vi "RoboIME_UI.vi"(9 "Com UDP":T14={"UDP GrSim TX"=TRUE, "Address:"="192.168.37.12", "Port:"=10301}, 10 "RefBox UDP RX":T13={"Local IP:"="", "Server IP:"="224.5.23.1", "Port"="10003"}, 11 "SSL UDP RX":T13={"Local IP:"="", "Server IP:"="224.5.23.2", "Port"="10020"}) -> ()   [LabVIEW 2022 SP3]
uses:
  Vision_class/Old vision/Controls/Estimadores.ctl
  Vision_class/Old vision/Decode SSL and Refree Wrapper Package Folder/SSL Referee Game Status.ctl
  Vision_class/Old vision/Draw Field Folder/DrawTargets.ctl
  Vision_class/Old vision/Controls/SSL Field State.ctl
  Vision_class/Old vision/Controls/SSL Detection Frame.ctl
  Vision_class/Old vision/Controls/SSL Detection Robot.ctl
  <vilib>/Analysis/Matrix/Datatypes/RealMatrix.ctl
  Vision_class/Old vision/Controls/SSL Detection Ball.ctl
  Communication_class/Communication.lvclass
  Controls/ComUDP.ctl
  Controls/ComSerial.ctl
  Controls/ComSOS.ctl
  Controls/PhoenixParameters.ctl
  Play_class/PassReceiver.ctl
  Parameters_class/ChoosePassReceiver.ctl
  Game_class/Navigation/Controls/bangBangControlParameters.ctl
  Parameters_class/Project.ctl
  Controls/RobotModelTestState.ctl
  Game_class/VelocityPlanningTest/Controls/testMode.ctl
  Controls/RobotModelReplacementTest.ctl
  Controls/grSimReplacement.ctl
  Communication_class/Paths/grSim Packet Command UDP Test Folder/grSim/grSim RobotReplacement.ctl
  Communication_class/Paths/grSim Packet Command UDP Test Folder/grSim/grSim_BallReplacement.ctl
  Game_class/KickValueTest/KickValuetest.ctl
  Game_class/KickValueTest/KickValue.ctl
  Game_class/KickValueTest/BallValue.ctl
  Game_class/VelocityPlanningTest/Controls/velocityPlanningState.ctl
  Game_class/VelocityPlanningTest/Controls/trajectoryState.ctl
  5RobotsPassGamePlay_class/PassFinishBallVelConditionDegub.ctl
  5RobotsPassGamePlay_class/PassFinishReceiverDistanceToBallConditionDebug.ctl
  Controls/Enviroment.ctl
  Team_class/KeeperPlay.ctl
  Team_class/OffensivePlay.ctl
  Referee_class/command_interpreted.ctl
  Robot_class/roles.ctl
  Robot_class/tactics.ctl
  Team_class/DefensivePlay.ctl
  Controls/vision_control.ctl
  Game_class/KickForceTest/Controls/kickForceTestState.ctl
  Game_class/KickForceTest/Controls/KickForceEnum.ctl
  Game_class/Replay/ReplayControls.ctl
  Game_class/ParametersFromFile/ParametersFromFile.ctl
  Robot_class/robotDisplayFeedback.ctl
  Controls/NewParameters.ctl
  Utilities_class/Style.ctl
  Vision_class/Vision.lvclass
  Game_class/Game.lvclass
  RobotFeedback/RobotFeedback.lvclass/RobotFeedback.ctl
  Game_class/Game.lvclass/Game.ctl
  Referee_class/Referee.lvclass/Referee.ctl
  Team_class/Team.lvclass/Team.ctl
  Robot_class/Robot.lvclass/Robot.ctl
  Game_class/ParametersFromFile/MainGameConfigs.ctl
  Robot_class/Robot.lvclass
  Events_class/Events.lvclass
  RobotFeedback/Read id.vi
  RobotFeedback/Read dribblerContactToBall.vi
  Game_class/Write RobotsFeedback.vi
  Robot_class/Read id.vi
  Robot_class/Read role.vi
  Robot_class/Read tactic.vi
  Game_class/Read Referee.vi
  Game_class/Read KeeperTeam.vi
  Game_class/Read OffensiveTeam.vi
  Game_class/Read DefensiveTeam.vi
  Team_class/Read RobotRef.vi
  Team_class/Read DefensivePlay.vi
  Team_class/Read OffensivePlay.vi
  Team_class/Read KeeperPlay.vi
  Referee_class/Read command_interpreted.vi
  Game_class/Write TestTeam.vi
  Game_class/Write DefensiveTeam.vi
  Game_class/Read AllyRef.vi
  Team_class/Write RobotRef.vi
  Game_class/Write NavigationTeam.vi
  Game_class/Write EventsRef.vi
  Game_class/Write OffensiveTeam.vi
  Game_class/Write KeeperTeam.vi
  Ally_class/Ally.lvclass
  C:/Users/ebert/Documents/codes/SSL/repo/SSL_AI/Team_class/Team.lvclass
  RobotFeedback/commCAS.vi
  Referee_class/Referee.lvclass
  Playbook_class/Playbook.lvclass
  <vilib>/Analysis/Matrix/NI_Matrix.lvlib
  RobotFeedback/RobotFeedback.lvclass
panel:
  in  "1st Penalty Kick Force":dbl
  in  "Chip Kick Penalty":bool
  in  "Boolean":bool
  in  "PID gains Lateral":cluster{"(Kc)":dbl, "(Ki)":dbl, "(Kd)":dbl}={"(Kc)"=2.0, "(Ki)"=0.0, "(Kd)"=0.001}
  in  "robotAngles":dbl[](array[numeric])=[30.0, 150.0, 225.0, 315.0] format="%#_13g"
  out "LastOffensivePlays":T1[](array[typedef])
  out "FPS Read UPD by Cam":dbl
  out "DefenseAvoidArea":bool
  in  "AttackerAvoidArea":bool
  out "KeeperPlay":T2=enum."NormalGame"
  out "OffensivePlay":T1=enum."TestPlay"
  out "DefensivePlay":T3=enum."Halt"
  out "command_interpreted":T4=enum."Halt"
  out "robotFeedback":cluster{"id":u32, "dribblerContact":bool}[](array[cluster])
  in  "Life Time":dbl=3.0
  in  "timeToValidateBall":dbl=1.0
  in  "PID gains Angle To Turn":cluster{"(Kc)":dbl, "(Ki)":dbl, "(Kd)":dbl}={"(Kc)"=4.5, "(Ki)"=0.0, "(Kd)"=0.001}
  in  "Line?":bool
  in  "BallOut":bool
  out "replaceBall":bool
  out "replaceRobots":bool
  out "grSIM replacement":T5
  out "robotControlResponseConnectionID":refnum<k16>
  out "robotControlResponseErrorOut":errorcluster
  out "error out 2":errorcluster
  out "debugOffensivePlayFinished":T8[](array[typedef])
  out "passdebug":T9[](array[typedef])
  out "passFinishConditions":bool[](array[boolean])
  in  "Debug Ball":bool
  out "NaN?":bool
  out "Log":string
  out "Exit":i32
  in  "Args":string[](array[string])
  out "touch":bool
  in  "Field Size":T10
  in  "Debug":bool
  in  "ball velocity máx":dbl=8.0
  in  "PID gains Angle":cluster{"(Kc)":dbl, "(Ki)":dbl, "(Kd)":dbl}={"(Kc)"=4.5, "(Ki)"=0.0, "(Kd)"=0.001}
  in  "PID gains Vel D":cluster{"(Kp)":dbl, "(Ki)":dbl, "(Kd)":dbl}={"(Kp)"=0.25, "(Ki)"=0.1, "(Kd)"=0.001}
  in  "ChipKick activated":bool=TRUE
  out "error out":errorcluster
  in  "Draw Graphs":bool
  in  "Test":bool
  in  "Tab Control":T11(tab)
  in  "ParametersFromFile":T12
  in  "Com Serial":T15={"Serial TX"=FALSE, "Porta:"="COM12"}
  in  "Com SOS":T16={"UDP SOS TX "=FALSE, "SOS Port: 2"=10025, "SOS Port: "=10021, "SOS Address:"="192.168.0.101"}
  out "RefBox RX":bool
  in  "Defense\n stretch":i32=2000
  in  "Defense\n width":i32=1000
  in  "Team":enum16{"Azul", "Amarelo"}(ring) caption="Enum"
  in  "Side":enum16{"Esquerdo", "Direito"}(ring) caption="Enum"
  in  "Goalie":string(combo)="0"
  in  "Command":string(combo)="Auto"
  in  "AttakingOurselves":bool
  out "SSL RX":bool
  in  "FIRASim?":bool
  in  "Project":T17
  in  "Envirnoment":T18=enum."realGame"
  in  "ViewState":T19(ring)=enum."Maximized"
  out "RefBox RX 2":bool
  out "SSL RX":bool
  out "displayFeedbackRobot":T20[](array[typedef]) {"Battery (V)" scale=6.0..8.4}
  out "Side out":enum16{"Esquerdo", "Direito"}(ring) caption="Enum"
  out "Team out":enum16{"Azul", "Amarelo"}(ring) caption="Enum"
  out "Envirnoment out":T18=enum."grSim"
  in  "ReplayControls":T21={"Slide"=0.0, "Enable"=FALSE, "FPS"=300.0, "On"=FALSE, "Play"=FALSE, "CopyFile"=FALSE, "CopyFilePathRelativeToLogFolder"="teste1.txt", "ReadFromFile"=FALSE, "ReadPathRelativeToLogFolder"="teste1.txt", "FrameBufferSize"=100000.0, "Speed"=1.0} {"Slide" scale=0.0..10.0}
  out "Slide out":dbl(slide) scale=0.0..10.0
  out "Keeper Team":cluster{"id":i32, "role":T22, "tactic":T23}[](array[cluster])
  out "Offensive Team":cluster{"id":i32, "role":T22, "tactic":T23}[](array[cluster])
  out "Defensive Team":cluster{"id":i32, "role":T22, "tactic":T23}[](array[cluster])
  in  "TestMode IDS":dbl[](array[numeric])
  out "SSL Referee Game Status":T24 {"Time" format="%<%.3X %x>T"; "Blue Timeout Remaining" format="%<%M:%S>t"; "Yellow Timeout Remaining" format="%<%M:%S>t"; "Time Left" format="%<%M:%S>t"}
  out "FPS Offensive":dbl
  out "FPS SetParameters":dbl
  out "FPS Defensive":dbl
  out "FPS Keeper":dbl
  out "FPS Com":dbl
  out "FPS Draw Field":dbl
  out "FPS Graph":dbl
  out "FPS referee":dbl
  out "FPS vision":dbl
  out "FPS Events":dbl
  in  "zigzag Points":cluster{"x":dbl, "y":dbl, "Angle":dbl}[](array[cluster])=[{"x"=-500.0, "y"=-500.0, "Angle"=0.0}, {"x"=-500.0, "y"=500.0, "Angle"=0.0}, {"x"=500.0, "y"=500.0, "Angle"=0.0}, {"x"=-500.0, "y"=500.0, "Angle"=0.0}]
  in  "TestMode":bool
  in  "Tests":enum16{"zigzag", "goto"}(ring)
  in  "Offensive ids":dbl[](array[numeric])
  in  "Defensive ids":dbl[](array[numeric])
  out "FPS Navigation":dbl
  out "FPS Read UDP":dbl
  out "FPS getCam":dbl
  out "FPS grSimTest":dbl
  out "FPS RobotFeedback":dbl
  in  "feedbackId":u32=5
  out "FPS Debug":dbl
  out "FPS ViewState":dbl
  out "FPS ReplaceErForce":dbl
  out "FPS RRTOffensive":dbl
  out "FPS Replay":dbl
  in  "RobotModelFolder\nFrom RobotModel":string
  in  "grSimTest":bool
  out "RobotModelState":T25 {"progress" scale=0.0..100.0}
  in  "Test":T26=enum."VelocityPlanning"
  in  "Reaplacement Tests":T27={"grSIM replacement"={"robots"=[], "ball"={"x"=0.0, "y"=0.0, "vx"=0.0, "vy"=0.0}}, "replace active"=FALSE, "TestParameters"={"Start"=FALSE, "V_sent(not used\nmore)"=0.0, "id"=0, "Samples"=0.0, "V_sample"=0.0, "delta"=0.2}, "Dest_array"=[], "replaceBall"=FALSE, "ballVelocity"=0.0, "timeoutKick"=0.0, "KickValueTest"={"ForceValue"={"delta_kick"=10.0, "kick_min"=40.0, "kick_max"=70.0}, "BallValue"={"delta_ball"=1.0, "v_min_ball"=-5.0, "v_max_ball"=2.0}, "Samples"=10.0, "Start"=FALSE, "id"=0, "RobotStopKick"=FALSE}, "StateSpaceTestParameters"={"Start"=FALSE, "uMaxPos"=0.4, "frequency"=40, "Samples"=5000.0, "uMinPos"=-0.4, "holdingFrequency"=50.0, "uMaxAngle"=1.5, "uMinAngle"=-1.5, "id"=0.0}}
  out "velocityPlanningState":T31={"est_vel"=0.0, "dist_to_(Dest/L)"=0.0, "V0_model"=0.0, "max_dist_to_break"=0.0, "v_sent"=0.0, "traj_state"=enum."replace"}
  out "kickForceTestState":T33={"currentKickForce"=0.0, "targetBallVelocity"=0.0, "est_bal_vell"=0.0, "sample"=0.0, "state"=enum."ReplaceBall"}
  in  "ABORT!!!!!!!!!":bool
  in  "id 3":dbl
  in  "id 2":dbl
  in  "id 1":dbl
  out "Robot":cluster{"Modulo":dbl, "Modulo":dbl}(graph)
  out "Robot":cluster{"Modulo":dbl, "Modulo":dbl}(graph)
  out "Ball_z":cluster{dbl}(graph)
  out "Ball_vel":cluster{"Modulo":dbl}(graph)
  out "Robot 2":cluster{"Modulo":dbl, "Modulo":dbl}(graph)
  in  "AI Parameters":T35={"Defensive Marker"=enum."SecondMostDangerous", "TimeoutDistanceInX"=600.0, "TimeoutDistanceInY"=600.0, "DistanceForaStillBall"=0.0, "TouchDistance"=110.0, "AttackerFarback"=1500.0, "MinDistToKick"=200.0, "Type of Marker"=enum."Auto", "Type of Defense "=enum."Manmark", "PassAngle"=0.045, "KickRange"=60.0, "KickForce"=50.0, "KickEps"=0.05, "KickAngle"=1.0, "Force++"=1.5, "DistanceToKickingAngle"=150.0, "DistanceToBallOut"=600.0, "DistanceStop"=750.0, "DistanceBehindAttacker"=200.0, "Area"=enum."Square", "DistanceForPossession"=180.0, "DistanceToConsirerRobotArrive"=50.0, "DistanceToGoAroundBall"=60.0, "DistanceInFrontOfAttacker"=200.0, "TimeoutDistanceBetweenRobots"=300.0, "MaxOutputAngle"=3.0, "MaxOutputXY"=3.5, "MaxDeceleration"=1.0, "MaxControlIncrement"=1.0, "MaxAcceleration"=4.0, "AngularToleranceForPossession"=0.3, "MaxVelBallToBeginDuelist"=0.5, "ZigZagAngle"=0.0, "PID gains Vel"={"(Kc)"=0.1, "(Ti, min)"=0.0, "(Td, min)"=2.0}, "Number of Offensive"=enum."Auto", "Shoot Out?"=FALSE, "DefenseAvoidArea"=FALSE, "InvertKick"=[], "Simple Pass"=FALSE, "ShootOutForce"=25.0, "dtPosEstBall"=0.3, "AttkIgnoreBallObst"=2500.0, "BarrierDist"=130.0, "PassReceiver"=enum."Auto", "GoalieInFrontGoal"=90.0, "RollToPass"=FALSE, "PassReceiver"=enum."Auto", "OldRRT"=FALSE, "Dribbler"=TRUE, "VelNearBall"=2.0, "ChipKick Force"=50.0, "ForcePass\nInGame"=10.0, "bangBangParameters"={"MaxVSent"=4.0, "MaxVNorm"=4.0, "MaxVAng"=8.0, "VAngCircle"=3.0, "LBeginCircle"=300.0, "DistToDestOrientation"=400.0, "MaxVAngToTurn"=8.0, "AtkDistToDestOrientation"=3500.0, "KepperMaxVSent"=4.0, "VelNearEnemy"=1.5}, "BallVelToAbortPass"=1.5, "BallVelToFinishPass"=1.0, "minDistanceToPass"=1000.0, "dribbler_rpm"=1.0, "AttackerAngle\nToTurnInDegrees"=5.0, "AttackerAngle\nToShootInDegrees"=0.5, "distToActivateDibbler"=1000.0, "StopVelocity"=1.2, "timeoutToShoot"=10.0, "DistanceArea"=100.0, "MinDistanceEnemy\nToBallToMark"=750.0, "DisableStopAvoidArea"=FALSE}
  in  "Id camera\ninf dir":dbl=1.0
  in  "Id camera\ninf esq":dbl=3.0
  in  "Id camera\nsup dir":dbl
  in  "Id camera\nsup esq":dbl=2.0
  in  "ignore left?":bool
  in  "ignore rigth?":bool
  in  "Estimador":T39=enum."Kalman"
  in  "Draw Targets?":T40={"Attacker"=TRUE, "Striker"=TRUE, "Goalie"=TRUE, "Defender"=TRUE, "kick"=TRUE, "Est Ball"=TRUE, "Est Robot"=FALSE, "Path S"=FALSE, "Path C"=FALSE, "Dngr.Enemy"=TRUE, "2nd Striker"=TRUE}
  in  "Draw Field":bool=TRUE
  in  "NewParameters":T41={"PenaltyDistance"=1200.0, "DistanceAttackerToBackBall"=40.0, "Division"=enum."Div B", "DistanceToAvoidyEnemyRobot"=600.0, "BallPlacementDistance"=900.0, "DisatanceBehindBallToStealBall"=600.0, "MaxDistanceToPositionKickoff"=2000.0, "BlockEnemyTarget"=TRUE, "MaxStopVAng"=4.0, "DistanceMarkerToEnemy"=600.0, "IgnoreDribblerContact"=FALSE, "DistanceToBeginEnemyPosession"=400.0, "GoToBallWhenEnemyNotMoving"=TRUE, "EnemyDistanceToReduceVelocity"=500.0, "TurnOnEnemyDistanceToReduceVelocity"=TRUE, "EnemyDistanceToShootOutBall"=0.0, "DefenseKickBall"=TRUE, "MoreKickToGoal? (0-0.3)"=0.24, "ChipKickInEnemyField"=TRUE, "ShootOutRobotId"=5.0, "FieldLenghtDenominatorInShootOut"=3.4, "AdjustPositionInBallPlacement"=FALSE, "PowerGodPass"=0.75, "VelocityAbortEnemyPos"=3.0, "MaxDistToBeginPass"=300.0, "MinDistToBeginPass"=150.0, "VelocityInDirects"=0.3, "BadDribblerIDs"=[1, 2, 3, 4, 5], "NewKickToDistanceAroundBall"=300.0, "PowerAvoidColisionMarker"=1.0, "DistanceToAvoidColisionMarker"=0.0, "AvoidBallKick"=70.0, "DistanceTryKick"=-250.0, "SuicideKickDIstance"=80.0, "FirstKickAtck"=TRUE, "AdjustFirstKickDistance"=100.0, "FirstKickDefense"=FALSE, "AvoidAimLessKick"=0.7, "DistanceToAvoidyEnemyShootRobot "=100.0, "NumberOfMarkers"=1.0, "PotField"=TRUE, "PIDLateral"=TRUE, "MinDistanceFirstKickX"=100.0, "MinDistanceFirstKickY"=750.0, "FractionOfDistToTouchGround\nAfterChipKick"=0.7, "FractionOfKickxWhen\nComposedWithKickz"=0.7, "Style"=enum."Offensive", "MoveInTurnState"=TRUE, "DistFromEnemyToConsider\nMoveInTurnState"=400.0, "CascadePID"=TRUE, "TurnAroundParameters"={"Radius"=170.0, "Multiplier"=2.0, "ChordAngle"=100.0}, "SafeDriveVel"=0.5, "DistanceToGoToBackBall"=500.0, "minDistanceToNotFinishEnemyPossession"=100.0, "Probability to kick direct penalty (0 - 1)"=0.0}
  in  "Communication in":refnum<class "Communication.lvclass">
  in  "Frame and Field Size out Ref":T43 {"Detection Frame Out"."robots_blue"."height" format="%+4.3f"; "Detection Frame Out"."robots_blue"."pixel_y" format="%+4.3f"; "Detection Frame Out"."robots_blue"."pixel_x" format="%+4.3f"; "Detection Frame Out"."robots_blue"."orientation" format="%+4.3f"; "Detection Frame Out"."robots_blue"."y" format="%+4.3f"; "Detection Frame Out"."robots_blue"."confidence" format="%4.3f"; "Detection Frame Out"."robots_blue"."x" format="%+4.3f"; "Detection Frame Out"."robots_yellow"."height" format="%+4.3f"; "Detection Frame Out"."robots_yellow"."pixel_y" format="%+4.3f"; "Detection Frame Out"."robots_yellow"."pixel_x" format="%+4.3f"; "Detection Frame Out"."robots_yellow"."orientation" format="%+4.3f"; "Detection Frame Out"."robots_yellow"."y" format="%+4.3f"; "Detection Frame Out"."robots_yellow"."confidence" format="%4.3f"; "Detection Frame Out"."robots_yellow"."x" format="%+4.3f"}
  out "2D Picture":picture
  in  "SSL Referee Game Status Ref":T24 {"Time" format="%<%.3X %x>T"; "Blue Timeout Remaining" format="%<%M:%S>t"; "Yellow Timeout Remaining" format="%<%M:%S>t"; "Time Left" format="%<%M:%S>t"}
  out "GUI Game Status":T24 {"Time" format="%<%.3X %x>T"; "Blue Timeout Remaining" format="%<%M:%S>t"; "Yellow Timeout Remaining" format="%<%M:%S>t"; "Time Left" format="%<%M:%S>t"}
  # "To execute Test and TestMode(zigzag)\nthe referee command must be Stop"
  # "PID gains vel:\nmakes the estimated velocity\ngoes closer into the desired velocity"
  # "Score"
  # "Red Cards"
  # "Yellow Cards"
  # "Timeouts Left"
  # "Timeout Remaining"
  # "Goalie ID"
  # "left goal"
  # "right goal"
  # "vision computer"
  # "Score"
  # "Red Cards"
  # "Yellow Cards"
  # "Timeouts Left"
  # "Timeout Remaining"
  # "Goalie ID"
  # "Score"
  # "Red Cards"
  # "Yellow Cards"
  # "Timeouts Left"
  # "Timeout Remaining"
  # "Goalie ID"
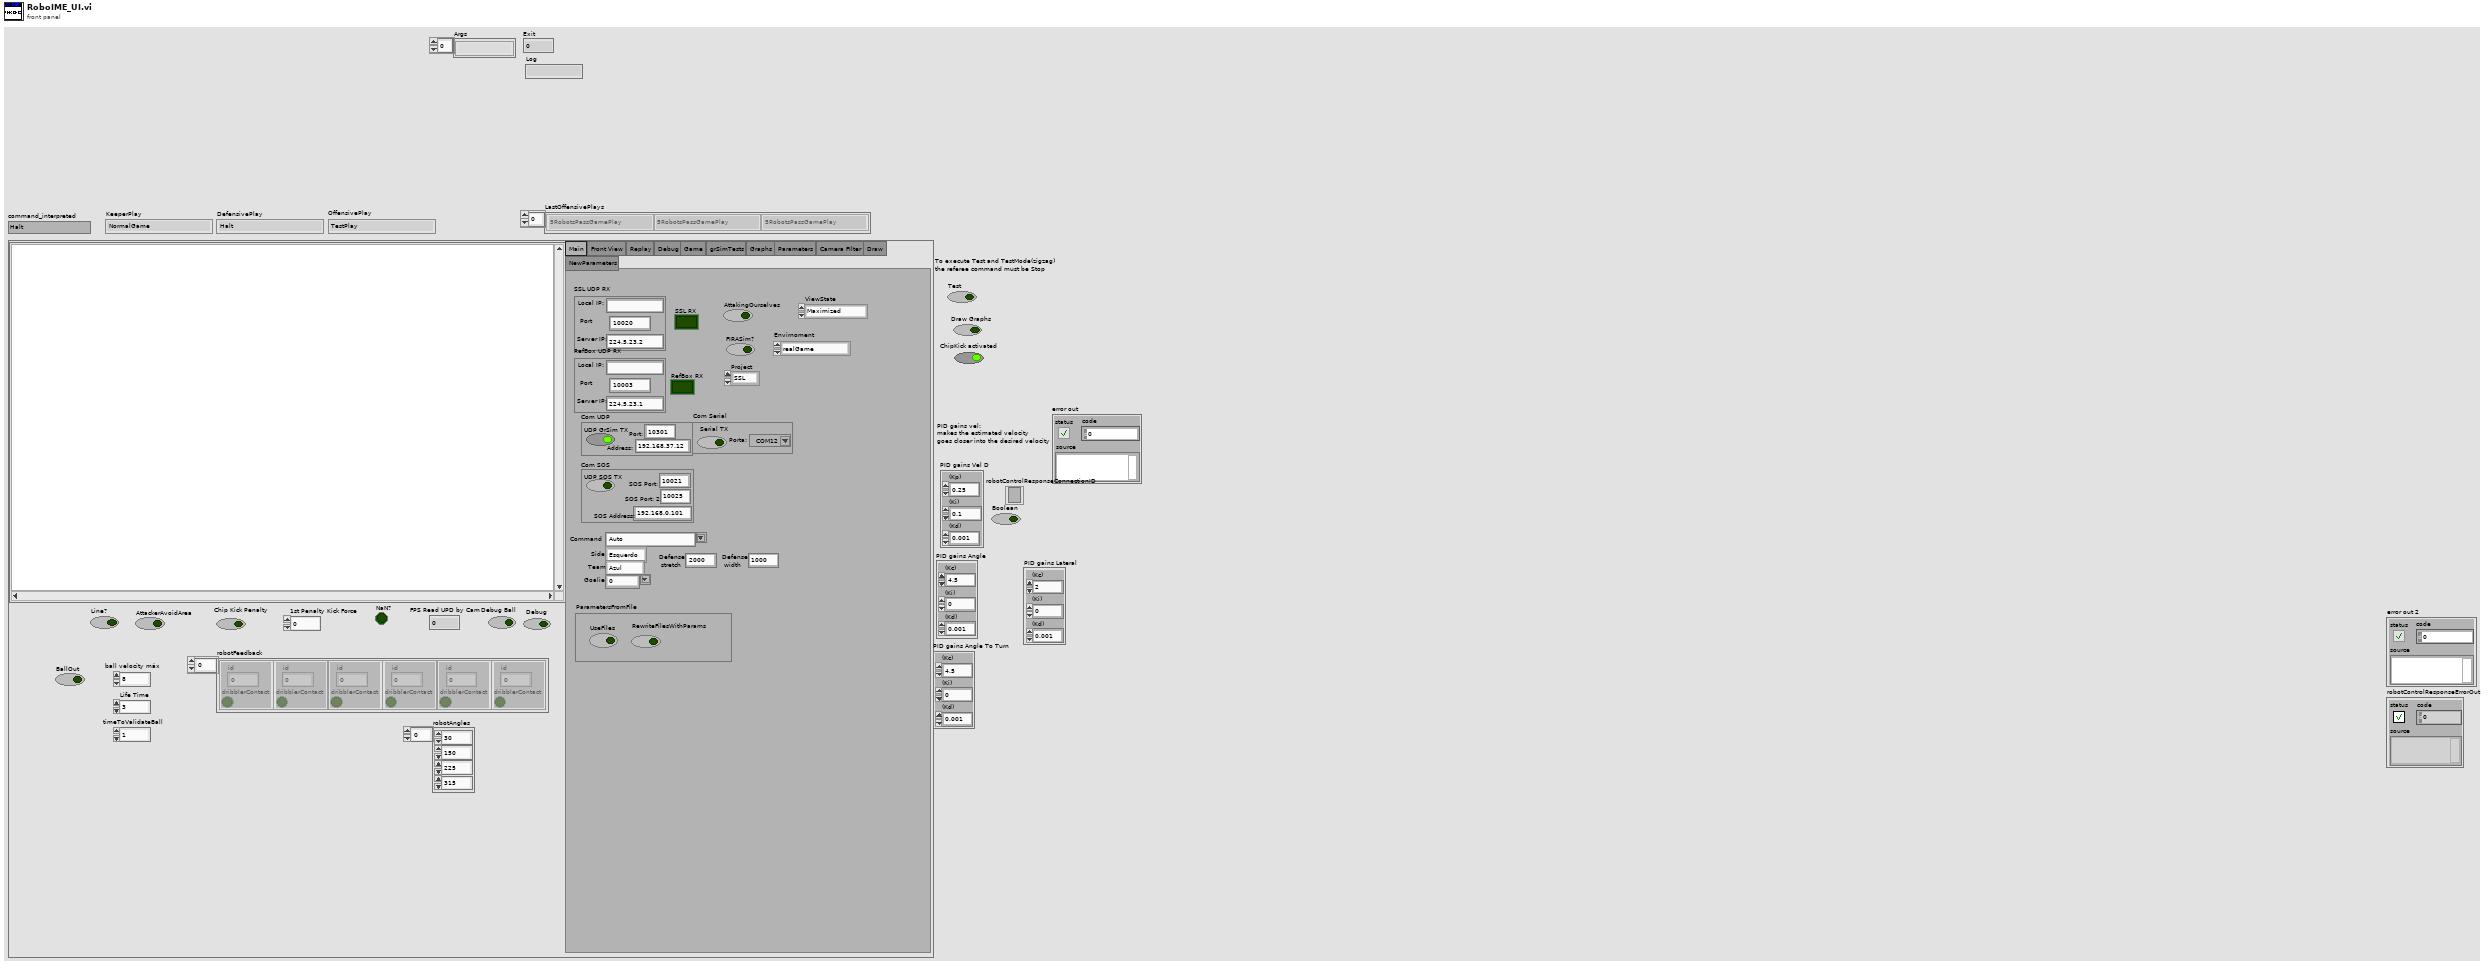
[diagram p1: front panel]
types:
  T1 = typedef "OffensivePlay.ctl" = enum16{"5RobotsPassGamePlay", "5PreparePassGame", "5RobotsKeeperGame", "KeeperPassToStriker", "5RobotsNormalGamePlay", "PrepareKeeperPass", "ACBPass", "ABCPass", "PrepareTriplePass", "TableWithStriker", "TableWith2ndStrikerPlay", "PrepareDoublePass", "PrepareRollToPass", "SimplePass", "PreparePass", "PassToStriker", "BallOutOfField", "PassTo2ndStriker", "StopOffensive", "Prepare Penalty Enemy", "EnemyPossessionAtEnemyField", "EnemyPossesionAtOurField", "TestPlay", "PreparePenaltyAlly", "KickPenaltyAlly", "PrepareKickoffAlly", "PrepareKickoffEnemy", "IndirectEnemy", "DirectEnemy", "PreparePassInGame1", "NormalGame", "DirectKick", "Pass", "Halt", "Timeout", "PassPlay", "PenaltyEnemy"}
  T2 = typedef "KeeperPlay.ctl" = enum16{"SimpleBallPlacementAlly", "BallPlacementAlly", "BallPlacementEnemy", "ZigZag", "Goto", "NormalGame", "KeeperPlay", "Halt", "Timeout", "PenaltyEnemy", "TestPlay"}
  T3 = typedef "DefensivePlay.ctl" = enum16{"NormalDefensiveWithDuelist", "NormalDefensive", "TestPlay", "Halt", "Timeout", "PenaltyEnemy", "PenaltyAlly"}
  T4 = typedef "command_interpreted.ctl" = enum16{"Goal Ally", "Goal Enemy", "Ball Placement Enemy", "Ball Placement Ally", "Normal Half Time", "Extra Time  Break", "Extra Half Time", "None", "Post Game", "PKA Normal Start", "Prepare Kickoff Ally", "PKE Normal Start", "Prepare Kickoff Enemy", "Force Start", "Halt", "Timeout", "Prepare Penalty Ally", "Prepare Penalty Enemy", "PPA NormalStart", "PPE Normal Start", "Indirect Free Ally", "Direct Free Enemy", "Direct Free Ally", "Indirect Free Enemy", "Stop"}
  T5 = typedef "grSimReplacement.ctl" = cluster{"robots":T6[], "ball":T7}
  T6 = typedef "grSim RobotReplacement.ctl" = cluster{"x":dbl, "y":dbl, "dir(degree)":dbl, "yellowteam":bool, "id":u32}
  T7 = typedef "grSim_BallReplacement.ctl" = cluster{"x":dbl, "y":dbl, "vx":dbl, "vy":dbl}
  T8 = typedef "PassFinishReceiverDistanceToBallConditionDebug.ctl" = cluster{"id_Receiver":i32, "ReceiverPosition":dbl[], "BallPosition":dbl[], "distanceBallToReceiver":dbl, "finish":bool}
  T9 = typedef "PassFinishBallVelConditionDegub.ctl" = cluster{"BallVel":dbl, "BallPosition":dbl[], "PasserPosition":dbl[], "distBallToPasser":dbl, "finished":bool, "vel_x":dbl, "vel_y":dbl}
  T10 = cluster{"line_width":u32, "field_length":u32, "field_width":u32, "boundary_width":u32, "referee_width":u32, "goal_width":u32, "goal_depth":u32, "goal_wall_width":u32, "center_circle_radius":u32, "defense_radius":u32, "defense_stretch":u32, "free_kick_from_defense_dist":u32, "penalty_spot_from_field_line_dist":u32, "penalty_line_from_spot_dist":u32}
  T11 = enum32{"Main", "Front View", "Replay", "Debug", "Game", "grSimTests", "Graphs", "Parameters", "Camera FIlter", "Draw", "NewParameters"}
  T12 = typedef "ParametersFromFile.ctl" = cluster{"UseFiles":bool, "RewriteFilesWithParams":bool}
  T13 = typedef "vision_control.ctl" = cluster{"Local IP:":string, "Server IP:":string, "Port":string}
  T14 = typedef "ComUDP.ctl" = cluster{"UDP GrSim TX":bool, "Address:":string, "Port:":u16}
  T15 = typedef "ComSerial.ctl" = cluster{"Serial TX":bool, "Porta:":refnum<visa-resource-name>}
  T16 = typedef "ComSOS.ctl" = cluster{"UDP SOS TX ":bool, "SOS Port: 2":u16, "SOS Port: ":u16, "SOS Address:":string}
  T17 = typedef "Project.ctl" = enum16{"SSL", "VSS"}
  T18 = typedef "Enviroment.ctl" = enum16{"erForceSimulator", "grSim", "realGame"}
  T19 = enum32{"Invalid", "Standard", "Closed", "Hidden", "Minimized", "Maximized"}
  T20 = typedef "robotDisplayFeedback.ctl" = cluster{"id":dbl, "encoder1":dbl, "encoder2":dbl, "kickCharge":bool, "ballInSensor":bool, "Battery (V)":dbl, "2D Picture":picture, "encoder3":dbl, "encoder4":dbl, "Valid":bool}
  T21 = typedef "ReplayControls.ctl" = cluster{"Slide":dbl, "Enable":bool, "FPS":dbl, "On":bool, "Play":bool, "CopyFile":bool, "CopyFilePathRelativeToLogFolder":string, "ReadFromFile":bool, "ReadPathRelativeToLogFolder":string, "FrameBufferSize":dbl, "Speed":dbl}
  T22 = typedef "roles.ctl" = enum16{"SimpleBallPlacement", "BallPlacementAllyPasser", "BallPlacementAllyReceiver", "BallPlacementEnemy", "5Robots5th", "PassBestReceiver", "5Robots4th", "5Robots3rd", "5Robots2nd", "5Robots1st", "PassBestRobot", "WaitPass", "ABCThirdKicker", "ABCFirstKicker", "ABCSecondKicker", "Tabler", "TableFinalizer", "PrepareRollToPassRoller", "PrepareRollToPassReceiver", "SimplePassRoll", "SimplePassRollReceiver", "PenaltyDefense", "PreparePassReceiver 2", "PreparePassReceiver 1", "PassObserver", "Timeout", "Goto", "ZigZag", "None", "BallOutOfField", "DefenderArea", "Duelist", "AttackerStop", "FollowAttacker", "KeeperRole", "KickPenalty", "AttackerAimGoal", "AttackerBlock", "Marker", "Halt", "Shoot", "PassKicker", "PassReceiver", "TestRole", "PenaltyAttacker"}
  T23 = typedef "tactics.ctl" = enum16{"GoToBallPlacementPosition", "PlaceBall", "GoToBallPlacement", "5Robots", "BallPlacementEnemy", "ReceivePassInFuturePoint", "Roller", "PrepareRollToPassRollerGoTo", "PrepareRollToPassReceiverGoTo", "WaitRoll", "PositionToRoll", "PenaltyAttacker", "PassObserver", "PenaltyDefense", "TableReceiverTactic", "Test", "DefendGoal", "Marker", "FollowAttacker", "DefendArea", "Shoot", "AttackerAimGoal", "AttackerBallOutOfField", "AttackerBlock", "AttackerStop", "Duelist", "Halt", "ZigZag", "GoTo", "Timeout", "KickToBestRobot", "KickToPassReceiver", "PositionToReceivePass", "WaitPass"}
  T24 = typedef "SSL Referee Game Status.ctl" = cluster{"Stage":string, "Command":string, "Time Left":dbl, "Yellow Team":string, "Blue Team":string, "Yellow Score":u32, "Blue Score":u32, "Yellow Red Cards":u32, "Blue Red Cards":u32, "Yellow Yellow Cards":u32, "Blue Yellow Cards":u32, "Yellow Timeouts Left":u32, "Blue Timeouts Left":u32, "Yellow Timeout Remaining":dbl, "Blue Timeout Remaining":dbl, "Yellow Goalie Id":u32, "Blue Goalie Id":u32, "Time":timestamp, "Point":cluster{"x":sgl, "y":sgl}}
  T25 = typedef "RobotModelTestState.ctl" = cluster{"current sample":i32, "V0":dbl, "Vf":dbl, "progress":dbl, "current state":i32, "est_vel":dbl, "V_sent":dbl, "crash cases":bool}
  T26 = typedef "testMode.ctl" = enum16{"KickForce", "ZigZag", "KickValue", "VelocityPlanning", "RobotModel", "RobotModelStateSpace", "CorumbaTest"}
  T27 = typedef "RobotModelReplacementTest.ctl" = cluster{"grSIM replacement":T5, "replace active":bool, "TestParameters":cluster{"Start":bool, "V_sent(not used\nmore)":dbl, "id":i32, "Samples":dbl, "V_sample":dbl, "delta":dbl}, "Dest_array":cluster{"dest_x":dbl, "dest_y":dbl, "dest_orientation":dbl, "dest_vel":dbl}[], "replaceBall":bool, "ballVelocity":dbl, "timeoutKick":dbl, "KickValueTest":T28, "StateSpaceTestParameters":cluster{"Start":bool, "uMaxPos":dbl, "frequency":i32, "Samples":dbl, "uMinPos":dbl, "holdingFrequency":dbl, "uMaxAngle":dbl, "uMinAngle":dbl, "id":dbl}}
  T28 = typedef "KickValuetest.ctl" = cluster{"ForceValue":T29, "BallValue":T30, "Samples":dbl, "Start":bool, "id":i32, "RobotStopKick":bool}
  T29 = typedef "Game.lvclass/KickValue.ctl" = cluster{"delta_kick":dbl, "kick_min":dbl, "kick_max":dbl}
  T30 = typedef "Game.lvclass/BallValue.ctl" = cluster{"delta_ball":dbl, "v_min_ball":dbl, "v_max_ball":dbl}
  T31 = typedef "velocityPlanningState.ctl" = cluster{"est_vel":dbl, "dist_to_(Dest/L)":dbl, "V0_model":dbl, "max_dist_to_break":dbl, "v_sent":dbl, "traj_state":T32}
  T32 = typedef "trajectoryState.ctl" = enum16{"stop", "replace", "circle", "line"}
  T33 = typedef "Game.lvclass/kickForceTestState.ctl" = cluster{"currentKickForce":dbl, "targetBallVelocity":dbl, "est_bal_vell":dbl, "sample":dbl, "state":T34}
  T34 = typedef "Game.lvclass/KickForceEnum.ctl" = enum16{"Finish", "Velball", "GoToNextKickForce", "WaitBall", "KickBall", "ReplaceBall"}
  T35 = typedef "PhoenixParameters.ctl" = cluster{"Defensive Marker":enum16{"SecondMostDangerous", "MostDangerous"}, "TimeoutDistanceInX":dbl, "TimeoutDistanceInY":dbl, "DistanceForaStillBall":dbl, "TouchDistance":dbl, "AttackerFarback":dbl, "MinDistToKick":dbl, "Type of Marker":enum16{"Auto", "BlockEnemyPass", "BlockOurGoal"}, "Type of Defense ":enum16{"Barreira", "Manmark"}, "PassAngle":dbl, "KickRange":dbl, "KickForce":dbl, "KickEps":dbl, "KickAngle":dbl, "Force++":dbl, "DistanceToKickingAngle":dbl, "DistanceToBallOut":dbl, "DistanceStop":dbl, "DistanceBehindAttacker":dbl, "Area":enum16{"Circular", "Square"}, "DistanceForPossession":dbl, "DistanceToConsirerRobotArrive":dbl, "DistanceToGoAroundBall":dbl, "DistanceInFrontOfAttacker":dbl, "TimeoutDistanceBetweenRobots":dbl, "MaxOutputAngle":dbl, "MaxOutputXY":dbl, "MaxDeceleration":dbl, "MaxControlIncrement":dbl, "MaxAcceleration":dbl, "AngularToleranceForPossession":dbl, "MaxVelBallToBeginDuelist":dbl, "ZigZagAngle":dbl, "PID gains Vel":cluster{"(Kc)":dbl, "(Ti, min)":dbl, "(Td, min)":dbl}, "Number of Offensive":enum16{"6", "5", "4", "3", "2", "1", "0", "Auto"}, "Shoot Out?":bool, "DefenseAvoidArea":bool, "InvertKick":dbl[], "Simple Pass":bool, "ShootOutForce":dbl, "dtPosEstBall":dbl, "AttkIgnoreBallObst":dbl, "BarrierDist":dbl, "PassReceiver":T36, "GoalieInFrontGoal":dbl, "RollToPass":bool, "PassReceiver":T37, "OldRRT":bool, "Dribbler":bool, "VelNearBall":dbl, "ChipKick Force":dbl, "ForcePass\nInGame":dbl, "bangBangParameters":T38, "BallVelToAbortPass":dbl, "BallVelToFinishPass":dbl, "minDistanceToPass":dbl, "dribbler_rpm":dbl, "AttackerAngle\nToTurnInDegrees":dbl, "AttackerAngle\nToShootInDegrees":dbl, "distToActivateDibbler":dbl, "StopVelocity":dbl, "timeoutToShoot":dbl, "DistanceArea":dbl, "MinDistanceEnemy\nToBallToMark":dbl, "DisableStopAvoidArea":bool}
  T36 = typedef "PassReceiver.ctl" = enum16{"Auto", "2ndStriker", "Striker"}
  T37 = typedef "ChoosePassReceiver.ctl" = enum16{"Striker", "2ndStriker", "Auto"}
  T38 = typedef "bangBangControlParameters.ctl" = cluster{"MaxVSent":dbl, "MaxVNorm":dbl, "MaxVAng":dbl, "VAngCircle":dbl, "LBeginCircle":dbl, "DistToDestOrientation":dbl, "MaxVAngToTurn":dbl, "AtkDistToDestOrientation":dbl, "KepperMaxVSent":dbl, "VelNearEnemy":dbl}
  T39 = typedef "Estimadores.ctl" = enum16{"Variable2ndDerivate", "4thDerivate", "2ndDerivate", "Nenhum", "Simples", "Kalman"}
  T40 = typedef "DrawTargets.ctl" = cluster{"Attacker":bool, "Striker":bool, "Goalie":bool, "Defender":bool, "kick":bool, "Est Ball":bool, "Est Robot":bool, "Path S":bool, "Path C":bool, "Dngr.Enemy":bool, "2nd Striker":bool}
  T41 = typedef "NewParameters.ctl" = cluster{"PenaltyDistance":dbl, "DistanceAttackerToBackBall":dbl, "Division":enum16{"Div B", "Div A"}, "DistanceToAvoidyEnemyRobot":dbl, "BallPlacementDistance":dbl, "DisatanceBehindBallToStealBall":dbl, "MaxDistanceToPositionKickoff":dbl, "BlockEnemyTarget":bool, "MaxStopVAng":dbl, "DistanceMarkerToEnemy":dbl, "IgnoreDribblerContact":bool, "DistanceToBeginEnemyPosession":dbl, "GoToBallWhenEnemyNotMoving":bool, "EnemyDistanceToReduceVelocity":dbl, "TurnOnEnemyDistanceToReduceVelocity":bool, "EnemyDistanceToShootOutBall":dbl, "DefenseKickBall":bool, "MoreKickToGoal? (0-0.3)":dbl, "ChipKickInEnemyField":bool, "ShootOutRobotId":dbl, "FieldLenghtDenominatorInShootOut":dbl, "AdjustPositionInBallPlacement":bool, "PowerGodPass":dbl, "VelocityAbortEnemyPos":dbl, "MaxDistToBeginPass":dbl, "MinDistToBeginPass":dbl, "VelocityInDirects":dbl, "BadDribblerIDs":i32[], "NewKickToDistanceAroundBall":dbl, "PowerAvoidColisionMarker":dbl, "DistanceToAvoidColisionMarker":dbl, "AvoidBallKick":dbl, "DistanceTryKick":dbl, "SuicideKickDIstance":dbl, "FirstKickAtck":bool, "AdjustFirstKickDistance":dbl, "FirstKickDefense":bool, "AvoidAimLessKick":dbl, "DistanceToAvoidyEnemyShootRobot ":dbl, "NumberOfMarkers":dbl, "PotField":bool, "PIDLateral":bool, "MinDistanceFirstKickX":dbl, "MinDistanceFirstKickY":dbl, "FractionOfDistToTouchGround\nAfterChipKick":dbl, "FractionOfKickxWhen\nComposedWithKickz":dbl, "Style":T42, "MoveInTurnState":bool, "DistFromEnemyToConsider\nMoveInTurnState":dbl, "CascadePID":bool, "TurnAroundParameters":cluster{"Radius":dbl, "Multiplier":dbl, "ChordAngle":dbl}, "SafeDriveVel":dbl, "DistanceToGoToBackBall":dbl, "minDistanceToNotFinishEnemyPossession":dbl, "Probability to kick direct penalty (0 - 1)":dbl}
  T42 = typedef "Style.ctl" = enum16{"Insanity", "Offensive", "Defensive"}
  T43 = typedef "SSL Field State.ctl" = cluster{"Detection Frame Out":T44, "Field Size Out":cluster{"line_width":u32, "field_length":u32, "field_width":u32, "boundary_width":u32, "referee_width":u32, "goal_width":u32, "goal_depth":u32, "goal_wall_width":u32, "center_circle_radius":u32, "defense_radius":u32, "defense_stretch":u32, "free_kick_from_defense_dist":u32, "penalty_spot_from_field_line_dist":u32, "penalty_line_from_spot_dist":u32}, "Received Time Stamp":timestamp}
  T44 = typedef "SSL Detection Frame.ctl" = cluster{"frame_number":u32, "t_capture":dbl, "t_sent":dbl, "camera_id":u32, "robots_yellow":T45[], "robots_blue":T45[], "balls":T47[], "Valid":bool, "Time Stamp":timestamp, "New":bool, "Initialized":bool}
  T45 = typedef "SSL Detection Robot.ctl" = cluster{"x":sgl, "robot_id":u32, "confidence":sgl, "y":sgl, "orientation":sgl, "pixel_x":sgl, "pixel_y":sgl, "height":sgl, "Valid":bool, "Time Stamp":timestamp, "x_k|k":T46, "Pk|k":T46, "Previous Time Stamp":timestamp, "R":T46, "vx":dbl, "vy":dbl, "vang":dbl}
  T46 = typedef "NI_Matrix.lvlib/RealMatrix.ctl" = dbl[][]
  T47 = typedef "SSL Detection Ball.ctl" = cluster{"x":sgl, "area":u32, "confidence":sgl, "y":sgl, "z":sgl, "pixel_x":sgl, "pixel_y":sgl, "Valid":bool, "Time Stamp":timestamp, "x_k|k":T46, "Pk|k":T46, "Id":u32, "Previous Time Stamp":timestamp, "R":T46, " vx":sgl, "vy":dbl, "vz":dbl, " ax":sgl, "ay":dbl, "az":dbl}
  T48 = typedef "ReplayInfo.ctl" = cluster{"ByteArrayFromVision":u8[], "TimeStampSampledInReplay":string, "ByteArrayFromReferee":u8[], "AllyRobotExtraInfoArray":T49[], "EnemyRobotExtraInfoArray":T49[]}
  T49 = typedef "RobotExtraInfo.ctl" = cluster{"est_vx":dbl, "est_vy":dbl, "id":dbl}
  T50 = typedef "AI Input.ctl" = cluster{"our_robots":T51[], "enemy_robots":T51[], "balls":T60[], "geometry":T61, "IA Judge":T62, "Received Timestamp":timestamp, "Events":T64}
  T51 = typedef "AI Robot.ctl" = cluster{"id":u32, "function":T52, "x":dbl, "y":dbl, "orientation":dbl, "v_tangent":dbl, "v_normal":dbl, "v_ang":dbl, "kick_x":dbl, "kick_z":dbl, "dribble":bool, "Timestamp":timestamp, "estimatives":T53, "dest_x_kick":dbl, "dest_y_kick":dbl, "Gap Coord":dbl[], "States":T54, "Path ":dbl[][], "Path  Smooth":dbl[][], "Dest":T55, "vx_desired":dbl, "vy_desired":dbl, "slowBehavior":bool, "VSSStates":T57, "robotKickState":T58, "role":T22, "x_k|k":T46, "driveMode":T59}
  T52 = typedef "Functions Enum.ctl" = enum16{"2nd Striker", "Attacker", "Goalie", "Defender", "Striker", "Goto 0", "Dummy", "Kicker", "ZigZag 0", "ZigZag 1", "ZigZag 2", "ZigZag 3", "ZigZag 4", "ZigZag 5", "ZigZag 6", "ZigZag 7", "ZigZag 8", ""}
  T53 = typedef "estimatives.ctl" = cluster{"est_v_tangent":dbl, "est_v_normal":dbl, "est_vx":dbl, "est_vy":dbl, "Pos Robot Est":dbl[], "est_v_ang":dbl}
  T54 = typedef "AttackerStates.ctl" = enum16{"Pass", "GoToTangent", "BallGetting", "GoToKick", ""}
  T55 = typedef "PathDests.ctl" = T56[]
  T56 = typedef "PathDest.ctl" = cluster{"dest_x":dbl, "dest_y":dbl, "dest_orientation":dbl, "dest_vel":dbl}
  T57 = typedef "VSSAttackerStates.ctl" = enum16{"Pass", "GoToTangent", "BallGetting", "GoToKick", "Rotate anti-clockwise", "Rotate Clockwise", ""}
  T58 = typedef "robotKickToStates.ctl" = enum16{"shootFromDirect", "avoidCollideBall", "goToBackBall", "none", "walk", "turn", "oldKickToShoot", "oldKickToGoToBackBall", "shoot"}
  T59 = typedef "driveMode.ctl" = enum16{"Fast", "SafeDrive"}
  T60 = typedef "AI Ball.ctl" = cluster{"x":dbl, "y":dbl, "timestamp":timestamp, "Vel_x":dbl, "Vel_y":dbl, "Pos Bola Est":dbl[], "Valid":bool, "z":dbl, "Vel_z":dbl, "Accel_x":dbl, "Accel_y":dbl}
  T61 = typedef "Field Size.ctl" = cluster{"line_width":u32, "field_length":u32, "field_width":u32, "boundary_width":u32, "referee_width":u32, "goal_width":u32, "goal_depth":u32, "goal_wall_width":u32, "center_circle_radius":u32, "defense_radius":u32, "defense_stretch":u32, "free_kick_from_defense_dist":u32, "penalty_spot_from_field_line_dist":u32, "penalty_line_from_spot_dist":u32}
  T62 = typedef "AI Judge.ctl" = cluster{"stage":string, "command":string, "our_goalie_id":dbl, "enemy_goalie_id":dbl, "command enum":T63, "Time":enum16{"Azul", "Amarelo"}, "Point":cluster{"x":sgl, "y":sgl}}
  T63 = typedef "Command Enum.ctl" = enum16{"Halt", "Stop", "Force Start", "PKA Normal Start", "Prepare Kickoff Ally", "PKE Normal Start", "Prepare Kickoff Enemy", "Prepare Penalty Ally", "PPA Normal Start", "Prepare Penalty Enemy", "PPE Normal Start", "Direct Free Enemy", "Direct Free Ally", "Indirect Free Enemy", "Indirect Free Ally", "Timeout Enemy", "Timeout Ally", "Goal Enemy", "Goal Ally", "Ball Placement Enemy", "Ball Placement Ally", "Normal Half Time", "Extra Time Break", "Extra Half Time", "None", "Post Game"}
  T64 = typedef "Events.ctl" = cluster{"Touch":bool, "Ball out":bool, "id touch":dbl, "Ball out of \nVision":bool, "Ball inside \nGoalie area":bool, "Robot not responding":bool, "Robots responding status":dbl[], "Enemy Ball \nPossession":bool, "Pass State":bool, "id end of pass":dbl, "Kick":bool, "Id ini Possession":dbl, "Ball Possesion":bool, "Id Possesion":dbl, "Direct Kick":bool, "2nd Strk Ativo":bool}
  T65 = typedef "MainGameConfigs.ctl" = cluster{"SSL UDP RX":T13, "RefBox UDP RX":T13, "Com UDP":T14, "Command":string, "Goalie":string, "Side":enum16{"Esquerdo", "Direito"}, "Team":enum16{"Azul", "Amarelo"}}
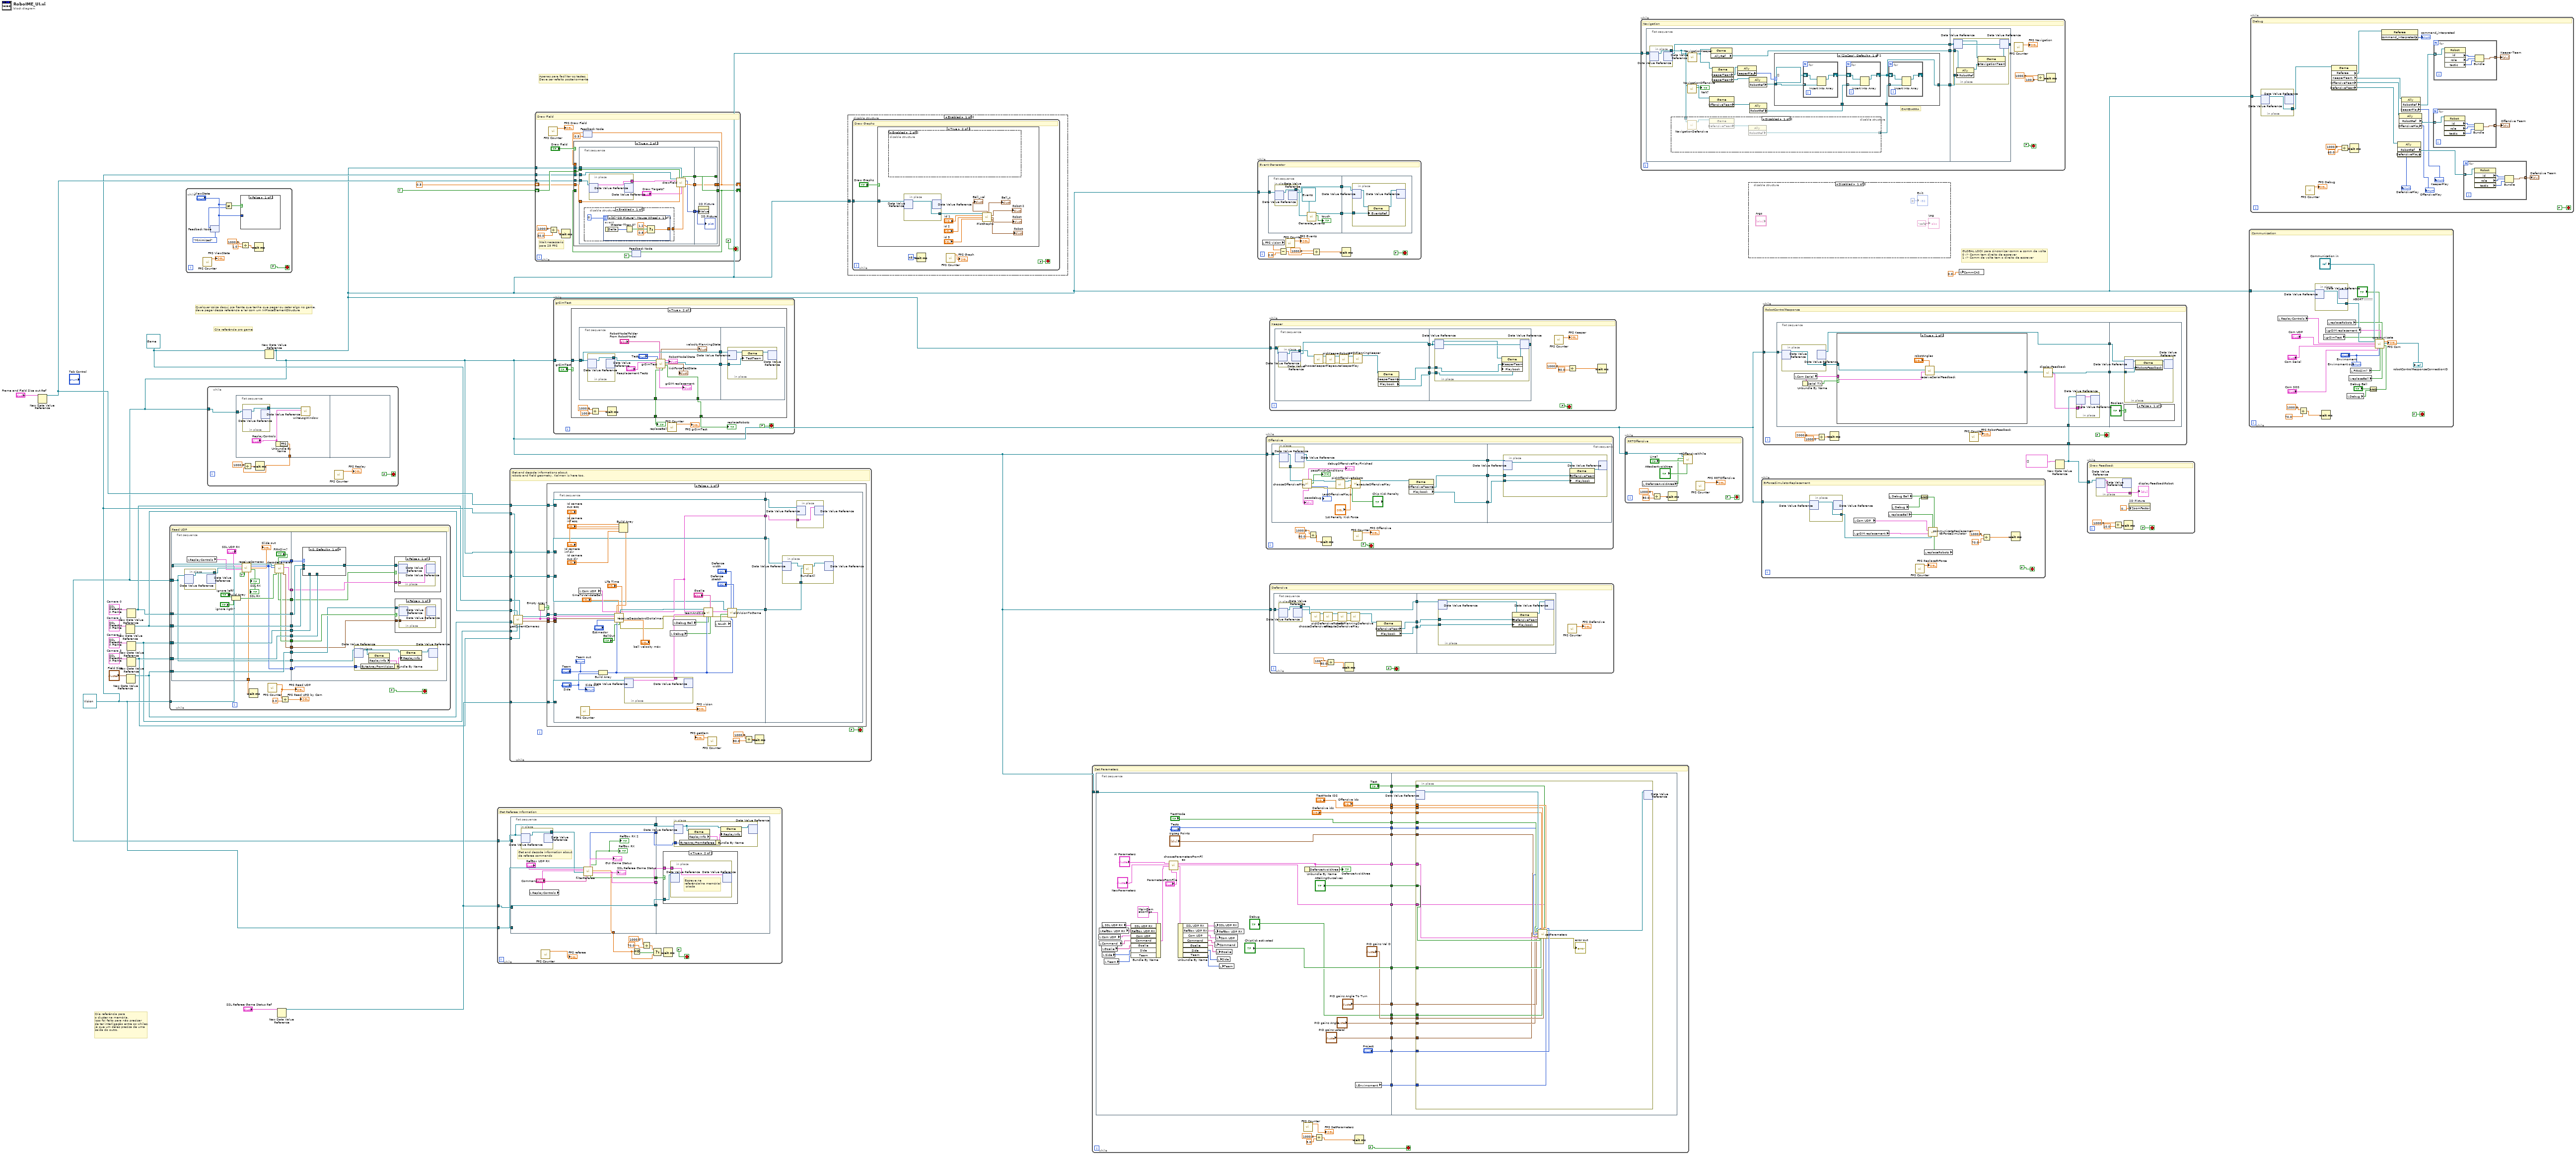
[diagram p0: block diagram]
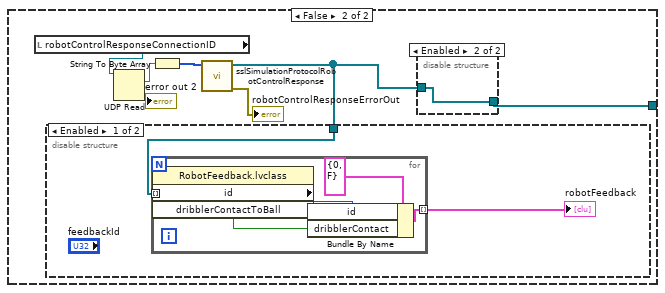
[diagram p9: hidden frame]
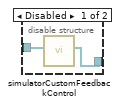
[diagram p10: hidden frame]
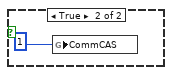
[diagram p12: hidden frame]
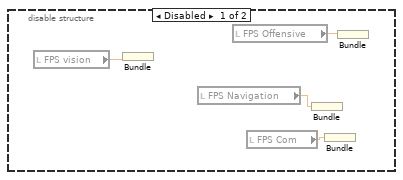
[diagram p17: hidden frame]
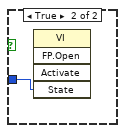
[diagram p19: hidden frame]
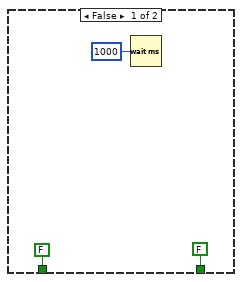
[diagram p20: hidden frame]
diagram:
  w11 = T44 {"frame_number"=0, "t_capture"=0.0, "t_sent"=0.0, "camera_id"=0, "robots_yellow"=[], "robots_blue"=[], "balls"=[], "Valid"=FALSE, "Time Stamp"=timestamp(0 s since 1904-01-01), "New"=FALSE, "Initialized"=FALSE}  # Camera 3
  w12 = T44 {"frame_number"=0, "t_capture"=0.0, "t_sent"=0.0, "camera_id"=0, "robots_yellow"=[], "robots_blue"=[], "balls"=[], "Valid"=FALSE, "Time Stamp"=timestamp(0 s since 1904-01-01), "New"=FALSE, "Initialized"=FALSE}  # Camera 2
  w13 = T44 {"frame_number"=0, "t_capture"=0.0, "t_sent"=0.0, "camera_id"=0, "robots_yellow"=[], "robots_blue"=[], "balls"=[], "Valid"=FALSE, "Time Stamp"=timestamp(0 s since 1904-01-01), "New"=FALSE, "Initialized"=FALSE}  # Camera 1
  w14 = T44 {"frame_number"=0, "t_capture"=0.0, "t_sent"=0.0, "camera_id"=0, "robots_yellow"=[], "robots_blue"=[], "balls"=[], "Valid"=FALSE, "Time Stamp"=timestamp(0 s since 1904-01-01), "New"=FALSE, "Initialized"=FALSE}  # Camera 0
  w16 = refnum<class "Game.lvclass"> refnum ("Game")
  w15 = refnum<class "Vision.lvclass"> refnum ("Vision")
  # "GLOBAL LOCK para sincronizar comm e comm de volta\n0 -> Comm tem direito de escrever\n1 -> Comm de volta tem o direito de escrever"
  # "Apenas para facilitar os testes.\nDeve ser refeito posteriormente"
  # "Qualquer coisa daqui pra frente que tenha que pegar ou setar algo no game,\ndeve pegar dessa referência e ler com um InPlaceElementStructure"
  # "Cria referência pro game"
  # "Cria referência para\no cluster na memória.\nIsso foi feito para não precisar\nde ter interligação entre os whiles,\njá que um deles precisa de uma\nsaída do outro."
  n1 = New Data Value Reference(data value="Frame and Field Size out Ref") -> (data value reference=w17:refnum<data-value>)  [unwired: 1 in, 1 out]
  n2 = New Data Value Reference(data value=w13) -> (data value reference=w6:refnum<data-value>)  [unwired: 1 in, 1 out]
  n3 = New Data Value Reference(data value="Field Size") -> (data value reference=w5:refnum<data-value>)  [unwired: 1 in, 1 out]
  n4 = New Data Value Reference(data value=w14) -> (data value reference=w7:refnum<data-value>)  [unwired: 1 in, 1 out]
  n5 = New Data Value Reference(data value=w12) -> (data value reference=w8:refnum<data-value>)  [unwired: 1 in, 1 out]
  n6 = New Data Value Reference(data value=w11) -> (data value reference=w9:refnum<data-value>)  [unwired: 1 in, 1 out]
  n7 = while {
    stop <- FALSE stop-if-true
    n8 = call "FPS Counter.vi"() -> ("FPS"=→"FPS ViewState":dbl)  [unwired: 11 in]
    n9 = feedback-in #1("ViewState") -> ()
    n10 = feedback #1(T19."Minimized" ("ViewState")) -> (w25:T19)
    n11 = Not Equal?(x="ViewState", y=w25) -> (x != y?=w24:bool)
    n12 = case shown="False" w24 {
      tunnel: "ViewState" -> [_ w32]
      frame False {
      }
      frame True {
        n13 = invoke class="VI" method="FP.Open"("State"=w32) -> ()  [unwired: 4 in, 5 out]
      }
    }
    n14 = Divide(x=1000.0, y=1.0) -> (x/y=w28:dbl)
    n15 = Wait (ms)(milliseconds to wait=w28) -> ()  [unwired: 1 out]
  }
  n16 = New Data Value Reference(data value=w16) -> (data value reference=w4:refnum<data-value>)  [unwired: 1 in, 1 out]
  n17 = while {
    tunnel: w15 -> [w56]
    tunnel: w5 -> [w55]
    tunnel: w9 -> [w53]
    tunnel: w7 -> [w51]
    tunnel: w6 -> [w49]
    tunnel: w8 -> [w47]
    tunnel: w4 -> [w37]
    stop <- FALSE stop-if-true
    # "Read UDP"
    n18 = flat-sequence {
      tunnel: w56 -> [w81]
      tunnel: w55 -> [w74]
      tunnel: [w79] -> w54
      tunnel: w53 -> [w79]
      tunnel: [w78] -> w52
      tunnel: w51 -> [w78]
      tunnel: [w77] -> w50
      tunnel: w49 -> [w77]
      tunnel: [w76] -> w48
      tunnel: w47 -> [w76]
      tunnel: [w75] -> w46
      tunnel: [w74] -> w45
      tunnel: [w73] -> w44
      tunnel: [w72] -> w43
      tunnel: [w66] -> w42
      tunnel: [w71] -> w41
      tunnel: w37 -> [w63]
      tunnel: [w63] -> w36
      tunnel: [w64] -> w35
      tunnel: [w60] -> w34
      tunnel: w54 -> [w92]
      tunnel: w52 -> [w95]
      tunnel: w50 -> [w94]
      tunnel: w48 -> [w93]
      tunnel: w46 -> [w90]
      tunnel: w45 -> [w89]
      tunnel: w44 -> [w88]
      tunnel: w43 -> [w87]
      tunnel: w42 -> [w86]
      tunnel: w41 -> [w85]
      tunnel: w36 -> [w84]
      tunnel: w35 -> [w83]
      frame #0 {
        n19 = in-place {
          in-place-border: [w82] -> w62
          n20 = in-place-dvr #2(w63) -> (w82:refnum<class "Game.lvclass">)  [unwired: 1 out]
          n21 = in-place-dvr #2() -> ()  [unwired: 1 in, 2 out]
        }
        n22 = local read "ReplayControls"() -> (w58:T21)
        n23 = Build Array("ignore left?", "ignore rigth?") -> (w68:bool[])
        n24 = call "receiveCameras.vi"("Vision in"=w81, "SSL UDP RX"="SSL UDP RX", "Game"=w62, "ReplayControls"=w58, "vision?"=TRUE) -> ("Vision out"=w80:refnum<class "Vision.lvclass">, "data camera out"=w64:u8[], "Slide out"=→"Slide out":dbl, "RX"=→"SSL RX" →"SSL RX":bool, "delay"=w60:dbl)  [unwired: 5 in, 1 out]
        n25 = call "decodeCameras.vi"("FIRASim?"="FIRASim?", "Ignore left/rigth?"=w68, "unsigned byte array"=w64, "Vision in"=w80) -> ("Field Size"=w73:T10, "Detection Frame"=w66:T44, "Empty Field Size?"=w75:bool, "camera_id"=w72:u32, "Empty Information?"=w71:bool)  [unwired: 1 in, 2 out]
      }
      frame #1 {
        n26 = case shown="0, Default" w87 {
          tunnel: [w96 w97 w98 w99] -> w91
          tunnel: w95 -> [w96 _ _ _]
          tunnel: w94 -> [_ w97 _ _]
          tunnel: w93 -> [_ _ w98 _]
          tunnel: w92 -> [_ _ _ w99]
          frame 0, Default {
          }
          frame 1 {
          }
          frame 2 {
          }
          frame 3 {
          }
        }
        n27 = in-place {
          in-place-border: w83 -> [w101]
          n28 = in-place-dvr #3(w84) -> (w103:refnum<class "Game.lvclass">)  [unwired: 1 out]
          n29 = property class="Game"(reference=w103) -> ("ReplayInfo"=w102:T48)  [unwired: 1 in, 2 out]
          n30 = Bundle By Name(cluster=w102, "ByteArrayFromVision"=w101) -> (w100:T48)
          n31 = property class="Game"(reference=w103, "ReplayInfo"=w100) -> (reference out=w104:refnum<class "Game.lvclass">)  [unwired: 1 in, 1 out]
          n32 = in-place-dvr #3(w104) -> ()  [unwired: 2 out]
        }
        n33 = case shown="False" w85 {
          tunnel: w91 -> [w109 _]
          tunnel: w86 -> [w108 _]
          frame False {
            n34 = in-place {
              in-place-border: w108 -> [w110]
              n35 = in-place-dvr #4(w109) -> ()  [unwired: 2 out]
              n36 = in-place-dvr #4(w110) -> ()  [unwired: 2 out]
            }
          }
          frame True {
          }
        }
        n37 = case shown="False" w90 {
          tunnel: w89 -> [w106 _]
          tunnel: w88 -> [w105 _]
          frame False {
            n38 = in-place {
              in-place-border: w105 -> [w107]
              n39 = in-place-dvr #5(w106) -> ()  [unwired: 2 out]
              n40 = in-place-dvr #5(w107) -> ()  [unwired: 2 out]
            }
          }
          frame True {
          }
        }
      }
    }
    n41 = Wait (ms)(milliseconds to wait=w34) -> ()  [unwired: 1 out]
    n42 = call "FPS Counter.vi"() -> ("FPS"=w40:dbl)  [unwired: 11 in]
    "FPS Read UDP" <- w40
    n43 = Divide(x=w40, y=4.0) -> (x/y=→"FPS Read UPD by Cam":dbl)
  }
  n44 = while {
    tunnel: w4 -> [w114]
    stop <- FALSE stop-if-true
    n45 = flat-sequence {
      tunnel: [w118] -> w111
      tunnel: w114 -> [w119]
      frame #0 {
        n46 = in-place {
          in-place-border: [w121] -> w120
          n47 = in-place-dvr #6(w119) -> (w121:refnum<class "Game.lvclass">)  [unwired: 1 out]
          n48 = in-place-dvr #6() -> ()  [unwired: 1 in, 2 out]
        }
        n49 = Unbundle By Name("ReplayControls") -> ("FPS"=w118:dbl)
        n50 = call "writeLogWindow.vi"("ReplayControls"="ReplayControls", "Game in"=w120) -> ()  [unwired: 8 in, 2 out]
      }
      frame #1 {
      }
    }
    n51 = Divide(x=1000.0, y=w111) -> (x/y=w116:dbl)
    n52 = Wait (ms)(milliseconds to wait=w116) -> ()  [unwired: 1 out]
    n53 = call "FPS Counter.vi"() -> ("FPS"=→"FPS Replay":dbl)  [unwired: 11 in]
  }
  n54 = New Data Value Reference(data value="SSL Referee Game Status Ref") -> (data value reference=w21:refnum<data-value>)  [unwired: 1 in, 1 out]
  n55 = while {
    tunnel: w15 -> [w137]
    tunnel: w21 -> [w133]
    tunnel: w4 -> [w127]
    stop <- FALSE stop-if-true
    # "Get Referee Information"
    n56 = flat-sequence {
      tunnel: w137 -> [w149]
      tunnel: [w147] -> w134
      tunnel: w133 -> [w147]
      tunnel: [w146] -> w132
      tunnel: [w144] -> w129
      tunnel: [w143] -> w128
      tunnel: w127 -> [w140]
      tunnel: [w142] -> w123
      tunnel: [w140] -> w126
      tunnel: w134 -> [w156]
      tunnel: w132 -> [w155]
      tunnel: w129 -> [w154]
      tunnel: w128 -> [w152]
      tunnel: w126 -> [w153]
      frame #0 {
        # "Get and decode information about\nde referee commands"
        n57 = in-place {
          in-place-border: [w151] -> w141
          n58 = in-place-dvr #7(w140) -> (w151:refnum<class "Game.lvclass">)  [unwired: 1 out]
          n59 = in-place-dvr #7() -> ()  [unwired: 1 in, 2 out]
        }
        n60 = local read "ReplayControls"() -> (w139:T21)
        n61 = call "filterReferee.vi"("Vision in"=w149, "RefBox UDP RX"="RefBox UDP RX", "ReplayControls"=w139, "Game"=w141, "Command"="Command") -> ("RX"=→"RefBox RX" →"RefBox RX 2":bool, "writeInReference"=w144:bool, "GUI Game Status"=→"GUI Game Status":T24, "delay"=w142:dbl, "SSL Referee Game Status"=w146:T24, "data camera out"=w143:u8[])  [unwired: 7 in, 2 out]
        "SSL Referee Game Status" <- w146
      }
      frame #1 {
        n62 = case shown="True" w154 {
          tunnel: w156 -> [_ w163]
          tunnel: w155 -> [_ w162]
          frame False {
          }
          frame True {
            n63 = in-place {
              in-place-border: w162 -> [w164]
              # "Escreve na\nreferência(na memória)\n criada"
              n64 = in-place-dvr #8(w163) -> ()  [unwired: 2 out]
              n65 = in-place-dvr #8(w164) -> ()  [unwired: 2 out]
            }
          }
        }
        n66 = in-place {
          in-place-border: w152 -> [w158]
          n67 = in-place-dvr #9(w153) -> (w160:refnum<class "Game.lvclass">)  [unwired: 1 out]
          n68 = property class="Game"(reference=w160) -> ("ReplayInfo"=w159:T48)  [unwired: 1 in, 2 out]
          n69 = Bundle By Name(cluster=w159, "ByteArrayFromReferee"=w158) -> (w157:T48)
          n70 = property class="Game"(reference=w160, "ReplayInfo"=w157) -> (reference out=w161:refnum<class "Game.lvclass">)  [unwired: 1 in, 1 out]
          n71 = in-place-dvr #9(w161) -> ()  [unwired: 2 out]
        }
      }
    }
    n72 = call "FPS Counter.vi"() -> ("FPS"=→"FPS referee":dbl)  [unwired: 11 in]
    n73 = Equal To 0?(x=w123) -> (x = 0?=w125:bool)
    n74 = Divide(x=1000.0, y=70.0) -> (x/y=w124:dbl)
    n75 = Select(t=w124, s=w125, f=w123) -> (s? t:f=w122:dbl)
    n76 = Wait (ms)(milliseconds to wait=w122) -> ()  [unwired: 1 out]
  }
  n77 = while {
    tunnel: w15 -> [w173]
    tunnel: w21 -> [w182]
    tunnel: w4 -> [w179]
    tunnel: w17 -> [w180]
    tunnel: w16 -> [w181]
    tunnel: w9 -> [w177]
    tunnel: w8 -> [w176]
    tunnel: w7 -> [w174]
    tunnel: w6 -> [w175]
    tunnel: w5 -> [w178]
    stop <- FALSE stop-if-true
    # "Get and decode informations about\nrobots and field geometry. Kalman is here too."
    n78 = call "getCurrentCameras.vi"("Camera 3"=w177, "Camera 0"=w174, "Camera 2"=w176, "Camera 1"=w175, "Field Size"=w178, "Vision in"=w173) -> ("Field Size out"=w171:T10, "NewCameras"=w170:T44[], "Vision out"=w172:refnum<class "Vision.lvclass">)  [unwired: 2 in, 1 out]
    n79 = Empty Array?(array=w170) -> (empty?=w165:bool)
    n80 = case shown="False" w165 {
      tunnel: w182 -> [w190 _]
      tunnel: w181 -> [w189 _]
      tunnel: w180 -> [w188 _]
      tunnel: w179 -> [w187 _]
      tunnel: w170 -> [w186 _]
      tunnel: w172 -> [w185 _]
      tunnel: w171 -> [w184 _]
      frame False {
        n81 = flat-sequence {
          tunnel: w190 -> [w228]
          tunnel: w189 -> [w198]
          tunnel: w188 -> [w219]
          tunnel: w187 -> [w218]
          tunnel: [w195] -> w194
          tunnel: [w203] -> w193
          tunnel: [w219] -> w192
          tunnel: [w218] -> w191
          tunnel: w186 -> [w201]
          tunnel: w185 -> [w209]
          tunnel: w184 -> [w208]
          tunnel: w194 -> [w233]
          tunnel: w193 -> [w231]
          tunnel: w192 -> [w232]
          tunnel: w191 -> [w234]
          frame #0 {
            n82 = local read "Com UDP"() -> (w207:T14)
            n83 = call "FPS Counter.vi"() -> ("FPS"=→"FPS vision":dbl)  [unwired: 11 in]
            n84 = Build Array("Team", "Side") -> (w214:u16[])
            n85 = Build Array("Id camera\nsup esq", "Id camera\ninf esq", "Id camera\ninf dir", "Id camera\nsup dir") -> (w215:dbl[])
            n86 = call "receiveDecodeAndDoKalman.vi"("Vision in"=w209, "NewCameras"=w201, "Field Size"=w208, "Estimador"="Estimador", "cameras array"=w215, "team/side"=w214, "timeToValidateBall"="timeToValidateBall", "Com UDP"=w207, "BallOut"="BallOut", "Life Time"="Life Time", "max ball vel"="ball velocity máx") -> ("Vision out"=w212:refnum<class "Vision.lvclass">, "Frame and Field Size out"=w203:T43, "error out"=w213:errorcluster)  [unwired: 6 in]
            n87 = in-place {
              in-place-border: [w230] -> w229
              n88 = in-place-dvr #10(w228) -> (w230:T24)  [unwired: 1 out]
              n89 = in-place-dvr #10() -> ()  [unwired: 1 in, 2 out]
            }
            n90 = local read "Debug"() -> (w204:bool)
            n91 = local read "Debug Ball"() -> (w205:bool)
            n92 = call "teamAndSide.vi"("Vision in"=w212, "Goalie"="Goalie", "Field State Input"=w203, "Game Status"=w229, "error in (no error)"=w213, "team/side"=w214, "Debug Ball"=w205, "Debug"=w204) -> ("IA State"=w197:T50, "error out"=w196:errorcluster)  [unwired: 5 in, 1 out]
            n93 = local read "touch"() -> (w206:bool)
            n94 = call "oldVisionToGame.vi"("Defense stretch"="Defense\n stretch", "Team/ Side"=w214, "Defense width"="Defense\n width", "error in (no error)"=w196, "touch"=w206, "IA State"=w197, "Game in"=w198) -> ("Game out"=w195:refnum<class "Game.lvclass">)  [unwired: 3 in, 1 out]
            "Team out" <- "Team"
            "Side out" <- "Side"
          }
          frame #1 {
            n95 = in-place {
              in-place-border: w233 -> [w237]
              n96 = in-place-dvr #11(w234) -> (w238:refnum<class "Game.lvclass">)  [unwired: 1 out]
              n97 = call "BundleAll.vi"("Game in\nvision atualized"=w237, "Game in from reference"=w238) -> ("Game out"=w236:refnum<class "Game.lvclass">)  [unwired: 8 in, 1 out]
              n98 = in-place-dvr #11(w236) -> ()  [unwired: 2 out]
            }
            n99 = in-place {
              in-place-border: w231 -> [w235]
              n100 = in-place-dvr #12(w232) -> ()  [unwired: 2 out]
              n101 = in-place-dvr #12(w235) -> ()  [unwired: 2 out]
            }
          }
        }
      }
      frame True {
      }
    }
    n102 = call "FPS Counter.vi"() -> ("FPS"=→"FPS getCam":dbl)  [unwired: 11 in]
    n103 = Divide(x=1000.0, y=80.0) -> (x/y=w166:dbl)
    n104 = Wait (ms)(milliseconds to wait=w166) -> ()  [unwired: 1 out]
  }
  n105 = while {
    shift-right: [w247] -> _
    shift-left: 0.5 ("New Scale") -> [w254]
    shift-right: [w249] -> _
    shift-left: TRUE ("AutoScale Out") -> [w255]
    tunnel: w15 -> [w253]
    tunnel: w4 -> [w252]
    tunnel: w17 -> [w251]
    stop <- FALSE stop-if-true
    # "Wait necessario\npara 25 FPS"
    # "Draw Field"
    n106 = call "FPS Counter.vi"() -> ("FPS"=→"FPS Draw Field":dbl)  [unwired: 11 in]
    n107 = Divide(x=1000.0, y=30.0) -> (x/y=w241:dbl)
    n108 = Wait (ms)(milliseconds to wait=w241) -> ()  [unwired: 1 out]
    n109 = feedback #13(0.5 ("New Scale")) -> (w246:dbl)
    n110 = feedback #14(TRUE ("AutoScale Out")) -> (w248:bool)
    n111 = case shown="True" "Draw Field" {
      tunnel: [w256 w267] -> w247
      tunnel: [w257 w266] -> w249
      tunnel: w255 -> [_ w265]
      tunnel: w254 -> [_ w264]
      tunnel: w253 -> [_ w263]
      tunnel: w252 -> [_ w262]
      tunnel: w251 -> [_ w261]
      tunnel: w248 -> [w257 _]
      tunnel: w246 -> [w256 _]
      frame False {
      }
      frame True {
        n112 = flat-sequence {
          tunnel: w265 -> [w276]
          tunnel: w264 -> [w275]
          tunnel: w263 -> [w272]
          tunnel: w262 -> [w271]
          tunnel: w261 -> [w270]
          tunnel: [w278] -> w260
          tunnel: [w277] -> w259
          tunnel: [w268] -> w258
          tunnel: [w290] -> w266
          tunnel: [w291] -> w267
          tunnel: w260 -> [w291]
          tunnel: w259 -> [w290]
          tunnel: w258 -> [w289]
          frame #0 {
            n113 = disable-structure shown="Enabled" {
              disable-tunnel: [w280 1.0 ("Zoom")] -> w274
              frame Enabled {
                n114 = event shown="[0] \"2D Picture\": Mouse Wheel" {
                  selector: _ -> [_ _]
                  dyn-events: _ -> [_ _]
                  timeout: 0 -> [_ _]
                  tunnel: [w281 1.0] -> w280
                  event "2D Picture": Mouse Wheel {
                    n115 = event-data() -> ("Delta"=w285:i32)  [unwired: 1 in]
                    n116 = Greater Than 0?(x=w285) -> (x > 0?=w284:bool)
                    n117 = Select(t=1.2, s=w284, f=0.8) -> (s? t:f=w281:dbl)
                  }
                  event Timeout {
                    n118 = event-data() -> ()  [unwired: 1 in, 3 out]
                  }
                }
              }
              frame Disabled {
              }
            }
            n119 = in-place {
              in-place-border: [w288] -> w269
              n120 = in-place-dvr #15(w270) -> (w288:T43)  [unwired: 1 out]
              n121 = in-place-dvr #15() -> ()  [unwired: 1 in, 2 out]
            }
            n122 = call "drawField.vi"("Vision in"=w272, "AutoScale"=w276, "Game reference"=w271, "Field State Input"=w269, "Scale mm/pixel"=w275, "Draw Targets?"="Draw Targets?", "Zoom"=w274) -> ("AutoScale Out"=w277:bool, "2D Picture"=w268:picture, "Scale Out"=w278:dbl)  [unwired: 4 in, 2 out]
          }
          frame #1 {
            n123 = property on="2D Picture" class="Pict"("Value"=w289) -> ()  [unwired: 2 in, 2 out]
            "2D Picture" <- w289
          }
        }
      }
    }
    n124 = feedback-in #13(w247) -> ()
    n125 = feedback-in #14(w249) -> ()
  }
  n126 = while {
    tunnel: w4 -> [w297]
    stop <- FALSE stop-if-true
    # "grSimTest"
    n127 = case shown="True" "grSimTest" {
      tunnel: w297 -> [_ w306]
      tunnel: [FALSE ("replaceRobots") w302] -> w293
      tunnel: [FALSE ("replaceBall") w301] -> w292
      frame False {
        n128 = Wait (ms)(milliseconds to wait=u32 1000) -> ()  [unwired: 1 out]
      }
      frame True {
        n129 = flat-sequence {
          tunnel: w306 -> [w319]
          tunnel: [w319] -> w308
          tunnel: [w318] -> w307
          tunnel: [w312] -> w302
          tunnel: [w310] -> w301
          tunnel: w308 -> [w323]
          tunnel: w307 -> [w322]
          frame #0 {
            n130 = in-place {
              in-place-border: [w321] -> w320
              n131 = in-place-dvr #16(w319) -> (w321:refnum<class "Game.lvclass">)  [unwired: 1 out]
              n132 = in-place-dvr #16() -> ()  [unwired: 1 in, 2 out]
            }
            n133 = call "grSimTest.vi"("Game in"=w320, "RobotModelFolder"="RobotModelFolder\nFrom RobotModel", "Reaplacement Tests"="Reaplacement Tests", "Test"="Test") -> ("velocityPlanningState"=→"velocityPlanningState":T31, "State"=→"RobotModelState":T25, "TestTeam"=w318:refnum<class "Ally.lvclass">, "kickForceTestState"=→"kickForceTestState":T33, "replaceRobots"=w312:bool, "grSIM replacement"=→"grSIM replacement":T5, "replaceBall"=w310:bool)  [unwired: 3 in, 2 out]
          }
          frame #1 {
            n134 = in-place {
              in-place-border: w322 -> [w325]
              n135 = in-place-dvr #17(w323) -> (w326:refnum<class "Game.lvclass">)  [unwired: 1 out]
              n136 = property class="Game"(reference=w326, "TestTeam"=w325) -> (reference out=w324:refnum<class "Game.lvclass">)  [unwired: 1 in, 1 out]
              n137 = in-place-dvr #17(w324) -> ()  [unwired: 2 out]
            }
          }
        }
        n138 = Divide(x=1000.0, y=100.0) -> (x/y=w303:dbl)
        n139 = Wait (ms)(milliseconds to wait=w303) -> ()  [unwired: 1 out]
      }
    }
    "replaceRobots" <- w293
    "replaceBall" <- w292
    n140 = call "FPS Counter.vi"() -> ("FPS"=→"FPS grSimTest":dbl)  [unwired: 11 in]
  }
  n141 = disable-structure shown="Enabled" {
    disable-tunnel: w4 -> [w327 _]
    frame Enabled {
      n142 = while {
        tunnel: w327 -> [w331]
        stop <- FALSE stop-if-true
        # "Draw Graphs"
        n143 = case shown="True" "Draw Graphs" {
          tunnel: w331 -> [_ w342]
          frame False {
          }
          frame True {
            n144 = disable-structure shown="Enabled" {
              frame Disabled {
                n145 = local read "FPS vision"() -> (w347:dbl)
                n146 = Bundle("FPS vision"=w347) -> (w346:cluster{"FPS vision":dbl})  [unwired: 1 in]
                n147 = local read "FPS Navigation"() -> (w344:dbl)
                n148 = local read "FPS Offensive"() -> (w345:dbl)
                n149 = local read "FPS Com"() -> (w343:dbl)
                n150 = Bundle("FPS Navigation"=w344) -> ()  [unwired: 1 in, 1 out]
                n151 = Bundle("FPS Com"=w343) -> ()  [unwired: 1 in, 1 out]
                n152 = Bundle("FPS Offensive"=w345) -> ()  [unwired: 1 in, 1 out]
              }
              frame Enabled {
              }
            }
            n153 = in-place {
              in-place-border: [w348] -> w338
              n154 = in-place-dvr #18(w342) -> (w348:refnum<class "Game.lvclass">)  [unwired: 1 out]
              n155 = in-place-dvr #18() -> ()  [unwired: 1 in, 2 out]
            }
            n156 = call-dynamic "PlotGraphs.vi"("Game in"=w338, "id 1"="id 1", "id 2"="id 2", "id 3"="id 3") -> ("Ball_vel"=→"Ball_vel":cluster{"Modulo":dbl}, "Ball_z"=→"Ball_z":cluster{dbl}, "Robot 1"=→"Robot 2":cluster{"Modulo":dbl, "Modulo":dbl}, "Robot 2"=→"Robot":cluster{"Modulo":dbl, "Modulo":dbl}, "Robot 3"=→"Robot":cluster{"Modulo":dbl, "Modulo":dbl})  [unwired: 5 in, 2 out]
          }
        }
        n157 = Wait (ms)(milliseconds to wait=u32 45) -> ()  [unwired: 1 out]
        n158 = call "FPS Counter.vi"() -> ("FPS"=→"FPS Graph":dbl)  [unwired: 11 in]
      }
    }
    frame Disabled {
    }
  }
  n159 = while {
    tunnel: w4 -> [w372]
    stop <- FALSE stop-if-true
    # "Set Parameters"
    n160 = flat-sequence {
      tunnel: w372 -> [w402]
      tunnel: [w402] -> w368
      tunnel: ["Offensive ids"] -> w367
      tunnel: ["Defensive ids"] -> w366
      tunnel: ["zigzag Points"] -> w365
      tunnel: ["TestMode IDS"] -> w364
      tunnel: ["TestMode"] -> w363
      tunnel: ["Tests"] -> w362
      tunnel: ["Test"] -> w361
      tunnel: [w393] -> w360
      tunnel: ["AttakingOurselves"] -> w359
      tunnel: ["Debug"] -> w358
      tunnel: ["ChipKick activated"] -> w357
      tunnel: ["PID gains Vel D"] -> w356
      tunnel: ["PID gains Angle"] -> w355
      tunnel: ["PID gains Lateral"] -> w354
      tunnel: ["Project"] -> w353
      tunnel: ["PID gains Angle To Turn"] -> w351
      tunnel: [w392] -> w350
      tunnel: [w396] -> w349
      tunnel: w368 -> [w430]
      tunnel: w367 -> [w432]
      tunnel: w366 -> [w431]
      tunnel: w365 -> [w429]
      tunnel: w364 -> [w428]
      tunnel: w363 -> [w427]
      tunnel: w362 -> [w426]
      tunnel: w361 -> [w425]
      tunnel: w360 -> [w424]
      tunnel: w359 -> [w423]
      tunnel: w358 -> [w422]
      tunnel: w357 -> [w421]
      tunnel: w356 -> [w420]
      tunnel: w355 -> [w419]
      tunnel: w354 -> [w418]
      tunnel: w353 -> [w417]
      tunnel: w351 -> [w416]
      tunnel: w350 -> [w415]
      tunnel: w349 -> [w414]
      frame #0 {
        n161 = local read "Com UDP"() -> (w388:T14)
        n162 = local read "RefBox UDP RX"() -> (w389:T13)
        n163 = local read "Command"() -> (w387:string)
        n164 = local read "Goalie"() -> (w386:string)
        n165 = local read "SSL UDP RX"() -> (w390:T13)
        n166 = local read "Side"() -> (w385:enum16{"Esquerdo", "Direito"})
        n167 = local read "Team"() -> (w384:enum16{"Azul", "Amarelo"})
        n168 = Bundle By Name(cluster=T65 {"SSL UDP RX"={"Local IP:"="", "Server IP:"="224.5.23.2", "Port"="10020"}, "RefBox UDP RX"={"Local IP:"="", "Server IP:"="224.5.23.1", "Port"="10003"}, "Com UDP"={"UDP GrSim TX"=TRUE, "Address:"="172.29.47.23", "Port:"=10301}, "Command"="Force Start", "Goalie"="0", "Side"=enum."Esquerdo", "Team"=enum."Azul"} ("MainGameConfigs"), "SSL UDP RX"=w390, "RefBox UDP RX"=w389, "Com UDP"=w388, "Command"=w387, "Goalie"=w386, "Side"=w385, "Team"=w384) -> (w383:T65)
        n169 = call "chooseParametersFromFiles.vi"("AI Parameters"="AI Parameters", "NewParameters"="NewParameters", "MainGameConfigs"=w383, "ParametersFromFile"="ParametersFromFile") -> ("AI Parameters out"=w393:T35, "NewParameters out"=w392:T41, "MainGameConfigs out"=w382:T65)  [unwired: 11 in, 2 out]
        n170 = Unbundle By Name(w382) -> ("SSL UDP RX"=w381:T13, "RefBox UDP RX"=w380:T13, "Com UDP"=w379:T14, "Command"=w378:string, "Goalie"=w377:string, "Side"=w376:enum16{"Esquerdo", "Direito"}, "Team"=w375:enum16{"Azul", "Amarelo"})
        n171 = local write "SSL UDP RX"(w381) -> ()
        n172 = local write "RefBox UDP RX"(w380) -> ()
        n173 = local write "Command"(w378) -> ()
        n174 = local write "Com UDP"(w379) -> ()
        n175 = local write "Goalie"(w377) -> ()
        n176 = local write "Side"(w376) -> ()
        n177 = local write "Team"(w375) -> ()
        n178 = Unbundle By Name(w393) -> ("DefenseAvoidArea"=→"DefenseAvoidArea":bool)
        n179 = local read "Envirnoment"() -> (w396:T18)
      }
      frame #1 {
        n180 = in-place {
          in-place-border: w432 -> [w452]
          in-place-border: w431 -> [w451]
          in-place-border: w429 -> [w439]
          in-place-border: w428 -> [w449]
          in-place-border: w427 -> [w448]
          in-place-border: w426 -> [w447]
          in-place-border: w425 -> [w446]
          in-place-border: w424 -> [w445]
          in-place-border: w423 -> [w444]
          in-place-border: w422 -> [w442]
          in-place-border: w421 -> [w443]
          in-place-border: w420 -> [w441]
          in-place-border: w419 -> [w440]
          in-place-border: w418 -> [w437]
          in-place-border: w417 -> [w438]
          in-place-border: w416 -> [w435]
          in-place-border: w415 -> [w434]
          in-place-border: w414 -> [w433]
          n181 = in-place-dvr #19(w430) -> (w453:refnum<class "Game.lvclass">)  [unwired: 1 out]
          n182 = call "setParameters.vi"("Game in"=w453, "TestMode"=w448, "PID gains Lateral"=w437, "Tests"=w447, "PID gains Angle"=w440, "zigzag Points"=w439, "AI Parameters"=w445, "PID gains Angle To Turn"=w435, "Project"=w438, "AttakingOurselves"=w444, "Defensive ids"=w451, "ChipKick activated"=w443, "TestMode IDS"=w449, "Debug"=w442, "Offensive ids"=w452, "PID gains Vel D"=w441, "Test"=w446, "NewParameters"=w434, "Enviroment"=w433) -> ("Game out"=w450:refnum<class "Game.lvclass">, "error out"=→"error out":errorcluster)  [unwired: 7 in]
          n183 = in-place-dvr #19(w450) -> ()  [unwired: 2 out]
        }
      }
    }
    n184 = call "FPS Counter.vi"() -> ("FPS"=→"FPS SetParameters":dbl)  [unwired: 11 in]
    n185 = Divide(x=1000.0, y=5.0) -> (x/y=w369:dbl)
    n186 = Wait (ms)(milliseconds to wait=w369) -> ()  [unwired: 1 out]
  }
  n187 = while {
    tunnel: w4 -> [w463]
    stop <- FALSE stop-if-true
    # "Event Generator"
    n188 = local read "FPS vision"() -> (w456:dbl)
    n189 = flat-sequence {
      tunnel: w463 -> [w469]
      tunnel: [w466] -> w462
      tunnel: [w465] -> w461
      tunnel: w462 -> [w472]
      tunnel: w461 -> [w471]
      frame #0 {
        n190 = in-place {
          in-place-border: [w470] -> w468
          n191 = in-place-dvr #20(w469) -> (w470:refnum<class "Game.lvclass">)  [unwired: 1 out]
          n192 = in-place-dvr #20() -> (w466:refnum<data-value>)  [unwired: 1 in, 1 out]
        }
        n193 = call-dynamic "Generate_events.vi"("Game in"=w468, "Events in"=refnum<class "Events.lvclass"> refnum) -> ("touch"=→"touch":bool, "Events out"=w465:refnum<class "Events.lvclass">)  [unwired: 6 in, 2 out]
      }
      frame #1 {
        n194 = in-place {
          in-place-border: w471 -> [w474]
          n195 = in-place-dvr #21(w472) -> (w475:refnum<class "Game.lvclass">)  [unwired: 1 out]
          n196 = property class="Game"(reference=w475, "EventsRef"=w474) -> (reference out=w473:refnum<class "Game.lvclass">)  [unwired: 1 in, 1 out]
          n197 = in-place-dvr #21(w473) -> ()  [unwired: 2 out]
        }
      }
    }
    n198 = Subtract(x=w456, y=2.0) -> (x-y=w454:dbl)
    n199 = call "FPS Counter.vi"() -> ("FPS"=→"FPS Events":dbl)  [unwired: 11 in]
    n200 = Divide(x=1000.0, y=w454) -> (x/y=w457:dbl)
    n201 = Wait (ms)(milliseconds to wait=w457) -> ()  [unwired: 1 out]
  }
  n202 = while {
    tunnel: w4 -> [w483]
    stop <- FALSE stop-if-true
    # "Offensive"
    n203 = flat-sequence {
      tunnel: w483 -> [w500]
      tunnel: [w489] -> w482
      tunnel: [w495] -> w481
      tunnel: [w494] -> w480
      tunnel: w482 -> [w504]
      tunnel: w481 -> [w503]
      tunnel: w480 -> [w502]
      frame #0 {
        n204 = in-place {
          in-place-border: [w501] -> w493
          n205 = in-place-dvr #22(w500) -> (w501:refnum<class "Game.lvclass">)  [unwired: 1 out]
          n206 = in-place-dvr #22() -> (w494:refnum<data-value>)  [unwired: 1 in, 1 out]
        }
        n207 = call "chooseOffensivePlay.vi"("Game"=w493) -> ("error out"=w498:errorcluster, "passFinishConditions"=→"passFinishConditions":bool[], "Game out"=w497:refnum<class "Game.lvclass">, "passdebug"=→"passdebug":T9[], "debugOffensivePlayFinished"=→"debugOffensivePlayFinished":T8[], "Plays"=→"LastOffensivePlays":T1[])  [unwired: 5 in]
        n208 = call-dynamic "pickOffensiveRobots.vi"("error in (no error)"=w498, "Game in"=w497) -> ("error out"=w499:errorcluster, "Game out"=w496:refnum<class "Game.lvclass">)  [unwired: 8 in]
        n209 = call "executeOffensivePlay.vi"("error in (no error)"=w499, "Numeric"="1st Penalty Kick Force", "Chip Kick Penalty"="Chip Kick Penalty", "Game in"=w496) -> ("Game out"=w488:refnum<class "Game.lvclass">)  [unwired: 6 in, 1 out]
        n210 = property class="Game"(reference=w488) -> ("OffensiveTeam"=w489:refnum<class "Ally.lvclass">, "Playbook"=w495:refnum<class "Playbook.lvclass">)  [unwired: 1 in, 2 out]
      }
      frame #1 {
        n211 = in-place {
          in-place-border: w504 -> [w508]
          in-place-border: w503 -> [w507]
          n212 = in-place-dvr #23(w502) -> (w505:refnum<class "Game.lvclass">)  [unwired: 1 out]
          n213 = property class="Game"(reference=w505, "OffensiveTeam"=w508, "Playbook"=w507) -> (reference out=w506:refnum<class "Game.lvclass">)  [unwired: 1 in, 1 out]
          n214 = in-place-dvr #23(w506) -> ()  [unwired: 2 out]
        }
      }
    }
    n215 = Divide(x=1000.0, y=80.0) -> (x/y=w477:dbl)
    n216 = Wait (ms)(milliseconds to wait=w477) -> ()  [unwired: 1 out]
    n217 = call "FPS Counter.vi"() -> ("FPS"=→"FPS Offensive":dbl)  [unwired: 11 in]
  }
  n218 = while {
    tunnel: w4 -> [w516]
    stop <- FALSE stop-if-true
    # "Keeper"
    n219 = flat-sequence {
      tunnel: w516 -> [w524]
      tunnel: [w522] -> w515
      tunnel: [w521] -> w514
      tunnel: [w520] -> w513
      tunnel: [w533] -> _
      tunnel: w515 -> [w533]
      tunnel: w514 -> [w532]
      tunnel: w513 -> [w531]
      frame #0 {
        n220 = in-place {
          in-place-border: [w530] -> w518
          n221 = in-place-dvr #24(w524) -> (w530:refnum<class "Game.lvclass">)  [unwired: 1 out]
          n222 = in-place-dvr #24() -> (w522:refnum<data-value>)  [unwired: 1 in, 1 out]
        }
        n223 = call "chooseKeeperPlay.vi"("Game in"=w518) -> ("error out"=w528:errorcluster, "Game out"=w523:refnum<class "Game.lvclass">)  [unwired: 9 in]
        n224 = call "pickKeeperRobots.vi"("error in (no error)"=w528, "Game in"=w523) -> ("error out"=w529:errorcluster, "Game out"=w526:refnum<class "Game.lvclass">)  [unwired: 8 in]
        n225 = call "executeKeeperPlay.vi"("error in (no error)"=w529, "Game in"=w526) -> ("error out"=w527:errorcluster, "Game out"=w525:refnum<class "Game.lvclass">)  [unwired: 8 in]
        n226 = call-dynamic "pathPlanningKeeper.vi"("error in (no error)"=w527, "Game in"=w525) -> ("Game out"=w519:refnum<class "Game.lvclass">)  [unwired: 8 in, 1 out]
        n227 = property class="Game"(reference=w519) -> ("KeeperTeam"=w521:refnum<class "Ally.lvclass">, "Playbook"=w520:refnum<class "Playbook.lvclass">)  [unwired: 1 in, 2 out]
      }
      frame #1 {
        n228 = in-place {
          in-place-border: w532 -> [w535]
          in-place-border: w531 -> [w536]
          n229 = in-place-dvr #25(w533) -> (w534:refnum<class "Game.lvclass">)  [unwired: 1 out]
          n230 = property class="Game"(reference=w534, "KeeperTeam"=w535, "Playbook"=w536) -> (reference out=w537:refnum<class "Game.lvclass">)  [unwired: 1 in, 1 out]
          n231 = in-place-dvr #25(w537) -> ()  [unwired: 2 out]
        }
      }
    }
    n232 = call "FPS Counter.vi"() -> ("FPS"=→"FPS Keeper":dbl)  [unwired: 11 in]
    n233 = Divide(x=1000.0, y=80.0) -> (x/y=w511:dbl)
    n234 = Wait (ms)(milliseconds to wait=w511) -> ()  [unwired: 1 out]
  }
  n235 = while {
    tunnel: w4 -> [w545]
    stop <- FALSE stop-if-true
    # "Defensive"
    n236 = flat-sequence {
      tunnel: w545 -> [w558]
      tunnel: [w550] -> w544
      tunnel: [w549] -> w543
      tunnel: [w548] -> w542
      tunnel: w544 -> [w561]
      tunnel: w543 -> [w560]
      tunnel: w542 -> [w562]
      frame #0 {
        n237 = in-place {
          in-place-border: [w559] -> w551
          n238 = in-place-dvr #26(w558) -> (w559:refnum<class "Game.lvclass">)  [unwired: 1 out]
          n239 = in-place-dvr #26() -> (w548:refnum<data-value>)  [unwired: 1 in, 1 out]
        }
        n240 = call-dynamic "chooseDefensivePlay.vi"("Game in"=w551) -> ("error out"=w556:errorcluster, "Game out"=w557:refnum<class "Game.lvclass">)  [unwired: 9 in]
        n241 = call-dynamic "pickDefensiveRobots.vi"("error in (no error)"=w556, "Game in"=w557) -> ("error out"=w554:errorcluster, "Game out"=w555:refnum<class "Game.lvclass">)  [unwired: 8 in]
        n242 = call-dynamic "executeDefensivePlay.vi"("error in (no error)"=w554, "Game in"=w555) -> ("error out"=w553:errorcluster, "Game out"=w552:refnum<class "Game.lvclass">)  [unwired: 8 in]
        n243 = call-dynamic "pathPlanningDefensive.vi"("error in (no error)"=w553, "Game in"=w552) -> ("Game out"=w547:refnum<class "Game.lvclass">)  [unwired: 8 in, 1 out]
        n244 = property class="Game"(reference=w547) -> ("DefensiveTeam"=w550:refnum<class "Ally.lvclass">, "Playbook"=w549:refnum<class "Playbook.lvclass">)  [unwired: 1 in, 2 out]
      }
      frame #1 {
        n245 = in-place {
          in-place-border: w561 -> [w564]
          in-place-border: w560 -> [w565]
          n246 = in-place-dvr #27(w562) -> (w563:refnum<class "Game.lvclass">)  [unwired: 1 out]
          n247 = property class="Game"(reference=w563, "DefensiveTeam"=w564, "Playbook"=w565) -> (reference out=w566:refnum<class "Game.lvclass">)  [unwired: 1 in, 1 out]
          n248 = in-place-dvr #27(w566) -> ()  [unwired: 2 out]
        }
      }
    }
    n249 = Divide(x=1000.0, y=80.0) -> (x/y=w540:dbl)
    n250 = Wait (ms)(milliseconds to wait=w540) -> ()  [unwired: 1 out]
    n251 = call "FPS Counter.vi"() -> ("FPS"=→"FPS Defensive":dbl)  [unwired: 11 in]
  }
  n252 = while {
    tunnel: w4 -> [w569]
    stop <- FALSE stop-if-true
    # "RRTOffensive"
    n253 = local read "DefenseAvoidArea"() -> (w567:bool)
    n254 = Divide(x=1000.0, y=80.0) -> (x/y=w573:dbl)
    n255 = Wait (ms)(milliseconds to wait=w573) -> ()  [unwired: 1 out]
    n256 = call "rrtOffensiveWhile.vi"("AttackerAvoidArea"="AttackerAvoidArea", "Line?"="Line?", "Volta ao redor\nda área?"=w567, "GameReference in"=w569) -> ()  [unwired: 7 in, 1 out]
    n257 = call "FPS Counter.vi"() -> ("FPS"=→"FPS RRTOffensive":dbl)  [unwired: 11 in]
  }
  n258 = while {
    tunnel: w4 -> [w579]
    stop <- FALSE stop-if-true
    # "Navigation"
    n259 = flat-sequence {
      tunnel: [w598] -> w583
      tunnel: w579 -> [w597]
      tunnel: [w588] -> w578
      tunnel: [w591] -> w577
      tunnel: [w623] -> _
      tunnel: w583 -> [w623]
      tunnel: w578 -> [w622]
      tunnel: w577 -> [w621]
      frame #0 {
        # "GAMBIARRA"
        n260 = in-place {
          in-place-border: [w620] -> w599
          n261 = in-place-dvr #28(w597) -> (w620:refnum<class "Game.lvclass">)  [unwired: 1 out]
          n262 = in-place-dvr #28() -> (w598:refnum<data-value>)  [unwired: 1 in, 1 out]
        }
        n263 = disable-structure shown="Disabled" {
          disable-tunnel: w599 -> [w619 _]
          disable-tunnel: [w617 _] -> w595
          frame Disabled {
            n264 = call "NavigationDefensive.vi"("Game in"=w619) -> ("Game out"=w618:refnum<class "Game.lvclass">)  [unwired: 9 in, 1 out]
            n265 = property class="Game"(reference=w618) -> ("DefensiveTeam"=w616:refnum<class "Ally.lvclass">)  [unwired: 1 in, 2 out]
            n266 = property class="Ally"(reference=w616) -> ("RobotRef"=w617:refnum<class "Robot.lvclass">[])  [unwired: 1 in, 2 out]
          }
          frame Enabled {
          }
        }
        n267 = call "NavigationOffensive.vi"("Game in"=w599) -> ("NaN?"=→"NaN?":bool, "Game out"=w590:refnum<class "Game.lvclass">)  [unwired: 7 in, 2 out]
        n268 = call "NavigationKeeper.vi"("Game in"=w599) -> ("Game out"=w592:refnum<class "Game.lvclass">)  [unwired: 9 in, 1 out]
        n269 = property class="Game"(reference=w590) -> ("OffensiveTeam"=w593:refnum<class "Ally.lvclass">)  [unwired: 1 in, 2 out]
        n270 = property class="Game"(reference=w592) -> ("AllyRef"=w591:refnum<class "Ally.lvclass">)  [unwired: 1 in, 2 out]
        n271 = property class="Game"(reference=w592) -> ("KeeperTeam"=w587:refnum<class "Ally.lvclass">, "KeeperTeam"=w594:refnum<class "Ally.lvclass">)  [unwired: 1 in, 2 out]
        n272 = property class="Ally"(reference=w587) -> ("KeeperPlay"=w586:T2)  [unwired: 1 in, 2 out]
        n273 = property class="Ally"(reference=w594) -> ("RobotRef"=w596:refnum<class "Robot.lvclass">[])  [unwired: 1 in, 2 out]
        n274 = property class="Ally"(reference=w593) -> ("RobotRef"=w585:refnum<class "Robot.lvclass">[])  [unwired: 1 in, 2 out]
        n275 = case shown="\"ZigZag\", Default" w586 {
          tunnel: w596 -> [w605 w615]
          tunnel: w585 -> [w602 _]
          tunnel: w595 -> [w601 _]
          tunnel: [w600 w615] -> w588
          frame "ZigZag", Default {
            n276 = for {
              tunnel: w605 -> [w614] mode=indexing
              shift-right: [w612] -> w603
              shift-left: refnum<class "Robot.lvclass">[] [] -> [w613]
              n277 = Insert Into Array(array=w613, new element=w614) -> (w612:refnum<class "Robot.lvclass">[])  [unwired: 1 in]
            }
            n278 = for {
              tunnel: w602 -> [w611] mode=indexing
              shift-right: [w609] -> w600
              shift-left: w603 -> [w610]
              n279 = Insert Into Array(array=w610, new element=w611) -> (w609:refnum<class "Robot.lvclass">[])  [unwired: 1 in]
            }
            n280 = for {
              tunnel: w601 -> [w608] mode=indexing
              shift-right: [w606] -> _
              shift-left: w600 -> [w607]
              n281 = Insert Into Array(array=w607, new element=w608) -> (w606:refnum<class "Robot.lvclass">[])  [unwired: 1 in]
            }
          }
          frame "BallPlacementAlly" {
          }
        }
      }
      frame #1 {
        n282 = in-place {
          in-place-border: w622 -> [w627]
          in-place-border: w621 -> [w626]
          n283 = in-place-dvr #29(w623) -> (w625:refnum<class "Game.lvclass">)  [unwired: 1 out]
          n284 = property class="Ally"(reference=w626, "RobotRef"=w627) -> (reference out=w628:refnum<class "Ally.lvclass">)  [unwired: 1 in, 1 out]
          n285 = property class="Game"(reference=w625, "NavigationTeam"=w628) -> (reference out=w624:refnum<class "Game.lvclass">)  [unwired: 1 in, 1 out]
          n286 = in-place-dvr #29(w624) -> ()  [unwired: 2 out]
        }
      }
    }
    n287 = call "FPS Counter.vi"() -> ("FPS"=→"FPS Navigation":dbl)  [unwired: 11 in]
    n288 = Divide(x=1000.0, y=100.0) -> (x/y=w582:dbl)
    n289 = Wait (ms)(milliseconds to wait=w582) -> ()  [unwired: 1 out]
  }
  n290 = disable-structure shown="Disabled" {
    frame Disabled {
      "Exit" <- 0 ("Exit")
      "Log" <- "safe" ("Log")
    }
    frame Enabled {
    }
  }
  n291 = while {
    tunnel: w4 -> [w641]
    stop <- FALSE stop-if-true
    # "ErForceSimulatorReplacement"
    n292 = in-place {
      in-place-border: [w645] -> w631
      n293 = in-place-dvr #30(w641) -> (w645:refnum<class "Game.lvclass">)  [unwired: 1 out]
      n294 = in-place-dvr #30() -> ()  [unwired: 1 in, 2 out]
    }
    n295 = local read "grSIM replacement"() -> (w637:T5)
    n296 = local read "Com UDP"() -> (w638:T14)
    n297 = local read "replaceBall"() -> (w632:bool)
    n298 = local read "Debug Ball"() -> (w636:bool)
    n299 = local read "Debug"() -> (w635:bool)
    n300 = call "FPS Counter.vi"() -> ("FPS"=→"FPS ReplaceErForce":dbl)  [unwired: 11 in]
    n301 = And(x=w636, y=w635) -> (x .and. y?=w634:bool)
    n302 = local read "replaceRobots"() -> (w633:bool)
    n303 = call "communicateReplacementErForceSimulator.vi"("replaceBall"=w632, "degubBall"=w634, "Com UDP"=w638, "grSIM replacement"=w637, "Game"=w631, "replaceRobots"=w633) -> ()  [unwired: 8 in, 2 out]
    n304 = Divide(x=1000.0 ("y"), y=70.0) -> (x/y=w642:dbl)
    n305 = Wait (ms)(milliseconds to wait=w642) -> ()  [unwired: 1 out]
  }
  n306 = global write "commCAS.vi" "CommCAS"(0.0) -> ()
  n307 = New Data Value Reference(data value=T20[] [] ("displayFeedbackRobot 2")) -> (data value reference=w2:refnum<data-value>)  [unwired: 1 in, 1 out]
  n308 = while {
    tunnel: w4 -> [w651]
    tunnel: w2 -> [w647]
    stop <- FALSE stop-if-true
    # "RobotControlResponse"
    n309 = flat-sequence {
      tunnel: [w657] -> w652
      tunnel: w651 -> [w660]
      tunnel: [w662] -> w650
      tunnel: w647 -> [w656]
      tunnel: w652 -> [w689]
      tunnel: w650 -> [w688]
      frame #0 {
        n310 = in-place {
          in-place-border: [w665] -> w663
          n311 = in-place-dvr #31(w660) -> (w665:refnum<class "Game.lvclass">)  [unwired: 1 out]
          n312 = in-place-dvr #31() -> (w662:refnum<data-value>)  [unwired: 1 in, 1 out]
        }
        n313 = local read "Com Serial"() -> (w661:T15)
        n314 = Unbundle By Name(w661) -> ("Serial TX"=w659:bool)
        n315 = case shown="True" w659 {
          tunnel: [w666 w670] -> w658
          tunnel: w663 -> [w669 _]
          tunnel: w661 -> [w668 _]
          frame True {
            n316 = call "receiveSerialFeedback.vi"("robotAngles"="robotAngles", "Com Serial"=w668, "Game"=w669) -> ("RobotsFeedback"=w666:refnum<class "RobotFeedback.lvclass">[])  [unwired: 6 in, 2 out]
          }
          frame False {
            n317 = local read "robotControlResponseConnectionID"() -> (w672:refnum<k16>)
            n318 = UDP Read(connection ID=w672) -> (data out=w675:string, error out=→"error out 2":errorcluster)  [unwired: 3 in, 3 out]
            n319 = String To Byte Array(string=w675) -> (unsigned byte array=w674:u8[])
            n320 = call "sslSimulationProtocolRobotControlResponse.vi"("robotControlArray"=w674) -> ("error out"=→"robotControlResponseErrorOut":errorcluster, "RobotsFeedback"=w671:refnum<class "RobotFeedback.lvclass">[])  [unwired: 9 in]
            n321 = disable-structure shown="Enabled" {
              disable-tunnel: w671 -> [w681 _]
              frame Enabled {
                n322 = for {
                  tunnel: w681 -> [w684] mode=indexing
                  tunnel: [w685] -> w680 mode=indexing
                  n323 = property class="RobotFeedback.lvclass"(reference=w684) -> ("id"=w683:i32, "dribblerContactToBall"=w682:bool)  [unwired: 1 in, 2 out]
                  n324 = Bundle By Name(cluster=cluster{"id":u32, "dribblerContact":bool} {"id"=0, "dribblerContact"=FALSE} ("robotFeedback"), "id"=w683, "dribblerContact"=w682) -> (w685:cluster{"id":u32, "dribblerContact":bool})
                }
                "robotFeedback" <- w680
              }
              frame Disabled {
              }
            }
            n325 = disable-structure shown="Enabled" {
              disable-tunnel: w671 -> [w678 w679]
              disable-tunnel: [w677 w679] -> w670
              frame Disabled {
                n326 = call "simulatorCustomFeedbackControl.vi"("RobotsFeedback"=w678) -> ("feedback_array"=w677:refnum<class "RobotFeedback.lvclass">[])  [unwired: 8 in, 2 out]
              }
              frame Enabled {
              }
            }
          }
        }
        n327 = call "displayFeedback.vi"("feedback_array"=w658) -> ("robotDisplayFeedback"=w655:T20[], "feedback_array out"=w657:refnum<class "RobotFeedback.lvclass">[])  [unwired: 7 in, 2 out]
        n328 = in-place {
          in-place-border: w655 -> [w664]
          n329 = in-place-dvr #32(w656) -> ()  [unwired: 2 out]
          n330 = in-place-dvr #32(w664) -> ()  [unwired: 2 out]
        }
      }
      frame #1 {
        n331 = case shown="False" "Boolean" {
          frame False {
          }
          frame True {
            n332 = global write "commCAS.vi" "CommCAS"(1) -> ()
          }
        }
        n333 = in-place {
          in-place-border: w689 -> [w691]
          n334 = in-place-dvr #33(w688) -> (w693:refnum<class "Game.lvclass">)  [unwired: 1 out]
          n335 = property class="Game"(reference=w693, "RobotsFeedback"=w691) -> (reference out=w692:refnum<class "Game.lvclass">)  [unwired: 1 in, 1 out]
          n336 = in-place-dvr #33(w692) -> ()  [unwired: 2 out]
        }
      }
    }
    n337 = Divide(x=2000.0, y=1000.0) -> (x/y=w646:dbl)
    n338 = Wait (ms)(milliseconds to wait=w646) -> ()  [unwired: 1 out]
    n339 = call "FPS Counter.vi"() -> ("FPS"=→"FPS RobotFeedback":dbl)  [unwired: 11 in]
  }
  n340 = while {
    tunnel: w2 -> [w696]
    stop <- FALSE stop-if-true
    # "Draw Feedback"
    n341 = in-place {
      in-place-border: [w701] -> w695
      n342 = in-place-dvr #34(w696) -> (w701:T20[])  [unwired: 1 out]
      n343 = in-place-dvr #34() -> ()  [unwired: 1 in, 2 out]
    }
    "displayFeedbackRobot" <- w695
    n344 = Divide(x=1000.0, y=10.0) -> (x/y=w700:dbl)
    n345 = Wait (ms)(milliseconds to wait=w700) -> ()  [unwired: 1 out]
    n346 = property on="2D Picture" class="Pict"("ZoomFactor"=sgl 0.2 ("Zoom Factor")) -> ()  [unwired: 2 in, 2 out]
  }
  n347 = while {
    tunnel: w4 -> [w724]
    stop <- FALSE stop-if-true
    # "Communication"
    n348 = local read "ReplayControls"() -> (w703:T21)
    n349 = Divide(x=1000.0 ("y"), y=70.0) -> (x/y=w712:dbl)
    n350 = in-place {
      in-place-border: [w725] -> w716
      n351 = in-place-dvr #35(w724) -> (w725:refnum<class "Game.lvclass">)  [unwired: 1 out]
      n352 = in-place-dvr #35() -> ()  [unwired: 1 in, 2 out]
    }
    n353 = Wait (ms)(milliseconds to wait=w712) -> ()  [unwired: 1 out]
    n354 = local read "grSimTest"() -> (w715:bool)
    n355 = local read "grSIM replacement"() -> (w705:T5)
    n356 = local read "replaceRobots"() -> (w704:bool)
    n357 = local read "Debug"() -> (w709:bool)
    n358 = local read "replaceBall"() -> (w711:bool)
    n359 = local read "FIRASim?"() -> (w717:bool)
    n360 = And(x="Debug Ball", y=w709) -> (x .and. y?=w708:bool)
    n361 = call-dynamic "communicate.vi"("Communication in"="Communication in", "Game"=w716, "ReplayControls"=w703, "Com UDP"="Com UDP", "Com Serial"="Com Serial", "grSimTest"=w715, "Com SOS"="Com SOS", "ABORT"="ABORT!!!!!!!!!", "Enviroment"="Envirnoment", "grSIM replacement"=w705, "FIRASim?"=w717, "ReplaceRobots"=w704, "repalceBall"=w711, "Debug"=w708) -> ("Comm TX FPS"=→"FPS Com":dbl, "connection ID out"=→"robotControlResponseConnectionID":refnum<k16>)  [unwired: 2 in, 2 out]
    "Envirnoment out" <- "Envirnoment"
  }
  n362 = while {
    tunnel: w4 -> [w746]
    stop <- FALSE stop-if-true
    # "Debug"
    n363 = in-place {
      in-place-border: [w762] -> w731
      n364 = in-place-dvr #36(w746) -> (w762:refnum<class "Game.lvclass">)  [unwired: 1 out]
      n365 = in-place-dvr #36() -> ()  [unwired: 1 in, 2 out]
    }
    n366 = call "FPS Counter.vi"() -> ("FPS"=→"FPS Debug":dbl)  [unwired: 11 in]
    n367 = property class="Game"(reference=w731) -> ("Referee"=w737:refnum<class "Referee.lvclass">, "KeeperTeam"=w745:refnum<class "Ally.lvclass">, "OffensiveTeam"=w744:refnum<class "Ally.lvclass">, "DefensiveTeam"=w743:refnum<class "Ally.lvclass">)  [unwired: 1 in, 2 out]
    n368 = Divide(x=1000.0, y=60.0) -> (x/y=w730:dbl)
    n369 = Wait (ms)(milliseconds to wait=w730) -> ()  [unwired: 1 out]
    n370 = property class="Referee"(reference=w737) -> ("command_interpreted"=→"command_interpreted":T4)  [unwired: 1 in, 2 out]
    n371 = property class="Ally"(reference=w743) -> ("RobotRef"=w740:refnum<class "Robot.lvclass">[], "DefensivePlay"=→"DefensivePlay":T3)  [unwired: 1 in, 2 out]
    n372 = property class="Ally"(reference=w744) -> ("RobotRef"=w741:refnum<class "Robot.lvclass">[], "OffensivePlay"=→"OffensivePlay":T1)  [unwired: 1 in, 2 out]
    n373 = property class="Ally"(reference=w745) -> ("RobotRef"=w742:refnum<class "Robot.lvclass">[], "KeeperPlay"=→"KeeperPlay":T2)  [unwired: 1 in, 2 out]
    n374 = for {
      tunnel: w741 -> [w756] mode=indexing
      tunnel: [w753] -> w734 mode=indexing
      n375 = property class="Robot"(reference=w756) -> ("id"=w755:i32, "role"=w754:T22, "tactic"=w752:T23)  [unwired: 1 in, 2 out]
      n376 = Bundle("id"=w755, "role"=w754, "tactic"=w752) -> (w753:cluster{"id":i32, "role":T22, "tactic":T23})  [unwired: 1 in]
    }
    "Offensive Team" <- w734
    n377 = for {
      tunnel: w742 -> [w761] mode=indexing
      tunnel: [w758] -> w735 mode=indexing
      n378 = property class="Robot"(reference=w761) -> ("id"=w760:i32, "role"=w759:T22, "tactic"=w757:T23)  [unwired: 1 in, 2 out]
      n379 = Bundle("id"=w760, "role"=w759, "tactic"=w757) -> (w758:cluster{"id":i32, "role":T22, "tactic":T23})  [unwired: 1 in]
    }
    "Keeper Team" <- w735
    n380 = for {
      tunnel: w740 -> [w751] mode=indexing
      tunnel: [w748] -> w733 mode=indexing
      n381 = property class="Robot"(reference=w751) -> ("id"=w750:i32, "role"=w749:T22, "tactic"=w747:T23)  [unwired: 1 in, 2 out]
      n382 = Bundle("id"=w750, "role"=w749, "tactic"=w747) -> (w748:cluster{"id":i32, "role":T22, "tactic":T23})  [unwired: 1 in]
    }
    "Defensive Team" <- w733
  }
